vi "PH_Beamline.panel.vi"(0 "object ref":refnum<vi>, 5 "error in (no error)":errorcluster) -> (19 "error out":errorcluster)   [LabVIEW 2014, in "PH_Beamline.lvlib"]
doc: "By this VI a hardware switch can be monitored and switched. \n\nThe indicators \"FALSE\", \"TRUE\" and \"SWITCH STATE\" show the value of the Beckhoff-Tag: blue indicates bad tag status reference problems, darkgreen false and lightgreen true. If everything is working fine, \"FALSE\" and \"SWITCH STATE\" should show the same value, while \"TRUE\" has the opposite value. The caption of the sensors for \"FALSE\" and \"TRUE\" are taken out of the database. In case of only one or no sensor these GUI elements are not shown at all.\n\nThe oval button switches. It should be in the same state as the \"SWITCH STATE\" indicator. \n\n\"Delete Instance\" disconnects and removes the instance from the PCS.\n\n\nLicense Agreement for this software:\n\nCopyright (C)\nGesellschaft für Schwerionenforschung, GSI\nPlanckstr. 1\n64291 Darmstadt\nGermany\n\nContact: D.Beck@gsi.de \n\nThis program is free software; you can redistribute it and/or modify it under the terms of the GNU General Public License as published by the Free Software Foundation; either version 2 of the license, or (at your option) any later version.\n\nThis program is distributed in the hope that it will be useful, but WITHOUT ANYW ARRANTY; without even the implied warranty of MERCHANTABILITY or FITNESS FOR A PARTICULAR PURPOSE. See the GNU General License for more details (http://www.gnu.org).\n\nGesellschaft für Schwerionenforschung, GSI\nPlanckstr. 1, 64291 Darmstadt, Germany\nFor all questions and ideas contact: M.Richter@gsi.de, H.Brand@gsi.de or D.Beck@gsi.de.\nLast update: 18-DEC-2002"
uses:
  PH_Beamline.lvlib
  PH_Basics/PH_Common/Picture/PH_Picture.GUI Element 48x48.ctl
  PH_Basics/PH_Common/Picture/PH_Picture.GUI Element 36x36.ctl
  PH_Basics/PH_Common/Picture/PH_Picture.GUI Element 24x36.ctl
  PH_Basics/PH_Common/Picture/PH_Picture.GUI Element.ctl
  PH_Basics/PH_Common/Picture/PH_Picture.GUI Element 36x24.ctl
  PH_Basics/PH_Common/Picture/PH_Picture.GUI Element 60x12.ctl
  PH_Basics/PH_Common/Picture/PH_Picture.GUI Element 12x60.ctl
  PH_Beamline.Operation Mode.ctl
  PH_Beamline.Switch Instances.ctl
  PH_Beamline.6P Switch Instances.ctl
  PH_Beamline.Black Box Instances.ctl
  PH_Beamline.Switch GUI Instances.ctl
  PH_Beamline.Switch+6P Instances.ctl
  PH_Beamline.Force Sensor Instances.ctl
  PH_Basics/PH_SystemInformation/PH_SystemInformation.GUI Refs.ctl
  PH_BL-Master/PH_BL-Master.GUI Refs.ctl
  PH_Beamline.GUI Refs.ctl
  PH_Beamline.Motion GUI Instances.ctl
  PH_Basics/PH_StatusHandler/PH_StatusHandler.Status.ctl
  CS_Core/CSObj/CSObj.lvlib
  PH_Basics/PH_StatusHandler/PH_StatusHandler.lvlib
  PH_Basics/PH_Common/PH_Common.lvlib
  PH_Classes/PH_Switch/PH_Switch.lvlib
  PH_Motion/PH_Sixpack_Switch/PH_Sixpack_Switch.lvlib
  PH_Classes/PH_BlackBox/PH_BlackBox.lvlib
  PH_BL-Master/PH_BL-Master.lvlib
  PH_Basics/PH_SystemInformation/PH_SystemInformation.lvlib
  PH_Basics/PH_Class/PH_Class.lvlib
panel:
  in  "Force Sensor Instances":T1="MM1_ForceSensor"
  in  "Compressor_Turnbox_1_Trans_6PGUI":T2
  in  "Compressor_Turnbox_1_6PGUI":T3
  in  "Compressor_Turnbox_2_Trans_6PGUI":T2
  in  "Compressor_Turnbox_2_6PGUI":T3
  in  "Experiment_Targetmanipulator_6PGUI":T3
  in  "Experiment_Targetmanipulator_TRANS_6PGUI":T4
  in  "Experiment_Targetmanipulator_TURN_6PGUI":T3
  in  "Switch and 6P Instances":T5="BL_Position_MM5::MA_MM5_6PGUI"
  in  "Switch GUI Instances":T6="Shutter_Exp_Laserbay_Interlock"
  in  "Black Box Instances":T7="PA_CH1_BB"
  in  "6P Switch Instances":T8="COS_Sensitivity_Switch"
  in  "Switch Instances":T9="MA01_CH1"
  out "Exp.-Shutters closed":bool
  in  "Remote Desktop Connection":bool
  out "PHELIX_Beckhoff_Watchdog":bool caption="Failure Beckhoff"
  out "PHELIX_Timing_Mode":enum32{"10 Hz", "0.5 Hz", "Shot"}(radio) caption="Modeselector"
  out "Emergency Off":u32(colorbox)
  out "Igni FR: Heating off":bool
  out "Igni MA 5: Heating off":bool
  out "Igni MA 4: Heating off":bool
  out "Igni MA 3: Heating off":bool
  out "Igni MA 2: Heating off":bool
  out "Igni MA 1: Heating off":bool
  in  "Z6 Main":bool
  in  "PCS Main":bool
  in  "PCS System Indicator":bool
  in  "CoG":bool
  in  "Calibrator":bool
  in  "Image Statistician":bool
  out "Shutter_Exp3":bool=TRUE
  out "Shutter_Exp2":bool=TRUE
  out "Shutter_Exp1":bool=TRUE
  out "Shutter Exp 4 (Z6)":u32(colorbox)
  out "Shutter Exp 3":u32(colorbox)
  out "Shutter Exp 2":u32(colorbox)
  out "Shutter Exp 1":u32(colorbox)
  in  "Tab Control":T10(tab)=enum."In.-Box"
  in  "\"D:\\PCS\\Remote Access\\ns.rdp\"":bool caption="OK Button"
  out "ns Frontend ok":bool caption="ok"
  in  "ns_WP_RR_6PWpGUI":T11
  in  "Hop 15":bool
  out "BL ns 8":u32(colorbox)
  in  "NS_Shut_PA_BB":bool=TRUE
  out "BL ns 7":u32(colorbox)
  out "BL ns 6":u32(colorbox)
  out "BL ns 5":u32(colorbox)
  out "BL ns 4":u32(colorbox)
  out "BL ns 3":u32(colorbox)
  out "BL ns 2":u32(colorbox)
  out "BL ns 1":u32(colorbox)
  in  "ns_Nearfield_Ring_Exit_ImageOperator":bool=TRUE
  in  "ns_Nearfield_Ring_Exit_Cam":bool=TRUE
  in  "ns_Farfield_Ring_Exit_ImageOperator":bool=TRUE
  in  "ns_Farfield_Ring_Exit_Cam":bool=TRUE
  in  "ns_Exit_Powermeter":bool=TRUE
  in  "Hop 23":bool
  in  "\"D:\\PCS\\Remote Access\\fs.rdp\"":bool caption="OK Button"
  out "fs Frontend ok":bool caption="ok"
  out "BL fs 17":u32(colorbox)
  out "BL fs 16":u32(colorbox)
  in  "YLF_WP_6PWpGUI":T12
  in  "fs_WP_Exit_6PWpGUI":T11
  in  "fs_OO_Spectrometer":bool=TRUE
  out "BL fs 8":u32(colorbox)
  out "BL fs 10":u32(colorbox)
  in  "fs_RR_Cavity_NF2GUI":T3
  in  "fs_Stretcher_6PGUI":T3
  out "BL fs 15":u32(colorbox)
  in  "FS_Shut_PA_BB":bool=TRUE
  out "BL fs 14":u32(colorbox)
  in  "Hop 3":bool
  out "BL fs 13":u32(colorbox)
  in  "FS_Switch_YLF_BB":T3
  out "BL fs 12":u32(colorbox)
  out "BL fs 11":u32(colorbox)
  out "BL fs 7":u32(colorbox)
  out "BL fs 5":u32(colorbox)
  out "BL fs 9":u32(colorbox)
  out "BL fs 6":u32(colorbox)
  out "BL fs 4":u32(colorbox)
  out "BL fs 3":u32(colorbox)
  out "BL fs 2":u32(colorbox)
  out "BL fs 1":u32(colorbox)
  in  "fs_Nearfield_Frontend_ImageOperator":bool=TRUE
  in  "fs_Nearfield_Frontend_Cam":bool=TRUE caption="fs NF Exit Cam"
  in  "fs_Synchrolock_Watch":bool=TRUE
  out "uOPA ok":bool caption="ok"
  in  "\"D:\\PCS\\Remote Access\\uOPA.rdp\"":bool caption="OK Button"
  out "BL uOPA 9":u32(colorbox)
  in  "uOPA_Pump_OO_Spectrometer":bool=TRUE
  in  "uOPA_Pump_WP_6PWpGUI":T11
  out "BL uOPA 8":u32(colorbox)=6618880
  out "BL uOPA 7":u32(colorbox)
  out "BL uOPA 6":u32(colorbox)
  out "BL uOPA 5":u32(colorbox)
  out "BL uOPA 4":u32(colorbox)
  out "BL uOPA 3":u32(colorbox)
  out "BL uOPA 2":u32(colorbox)
  out "BL uOPA 1":u32(colorbox)
  out "BL uOPA 0":u32(colorbox)
  in  "Hop 24":bool
  in  "uOPA_Regen_Cam":bool=TRUE
  in  "uOPA_Pump_Powermeter":bool=TRUE
  in  "PA_SHS_Input_Cam":bool=TRUE
  in  "PA_CH1_BB":T13 caption="CH"
  out "BL PA 21":u32(colorbox)
  out "PA_Bypass_In":T3
  out "BL PA 24":u32(colorbox)
  out "BL PA 23":u32(colorbox)
  in  "PA_delayed_BB":bool=TRUE
  in  "PA_Input_2_Beam_6PWpGUI":T11
  out "BL PA 11":u32(colorbox)
  in  "PA_ML_T3_Exit_6P4QGUI":T11 caption="PA Lens"
  in  "PA_SA_6P4QGUI":T3
  out "BL PA 4":u32(colorbox)
  in  "PA_Input_Delay_6PGUI":T3
  out "BL PA 8":u32(colorbox)
  out "BL PA 7":u32(colorbox)
  out "BL PA 6":u32(colorbox)
  out "BL PA 5":u32(colorbox)
  out "BL PA 3":u32(colorbox)
  in  "PA_non_delayed_BB":bool=TRUE
  in  "PA-Backreflection-Meas":bool=TRUE
  in  "PA_PC_WP_2_BB":bool=TRUE
  in  "Hop 22":bool
  in  "Hop 16":bool
  out "BL PA 20":u32(colorbox)
  in  "PA_PC_WP_BB":bool=TRUE
  in  "PA_PiH_VSF2_6PGUI":T11
  out "BL PA 10":u32(colorbox)
  in  "PA_Shut_Input_BB":bool=TRUE
  in  "PA_PiH_VSF4_6PGUI":T11
  in  "Hop 6":bool
  in  "Hop 5":bool
  in  "Hop 4":bool
  in  "PA_MM_P_Input_NF2GUI":T3
  in  "PA_MM_C_Input_NF2GUI":T3
  out "BL PA 0":u32(colorbox)
  out "BL PA 16":u32(colorbox)
  out "BL PA 12":u32(colorbox)
  out "BL PA 14":u32(colorbox)
  out "PA_VacuumControl::PA_VacuumControl_Telescope 2":dbl=2000.0 caption="mbar" format="%#_2e"
  out "PA_VacuumControl::PA_VacuumControl_Telescope 3":dbl=2000.0 caption="mbar" format="%#_2e"
  out "PA_VacuumControl::PA_VacuumControl_Telescope 4":dbl=2000.0 caption="mbar" format="%#_2e"
  out "PA_VacuumControl::PA_VacuumControl_Bridge":dbl=2000.0 caption="mbar" format="%#_2e"
  out "BL PA 18":u32(colorbox)
  out "PA_Bypass_Out":T3
  out "BL PA 22":u32(colorbox)
  in  "PA_Switch_Lab_BB":T3
  in  "PA_Exit_Shut_BB":bool=TRUE
  out "BL PA 19":u32(colorbox)
  out "BL PA 15":u32(colorbox)
  out "BL PA 13":u32(colorbox)
  in  "PA_Nearfield_Input_ImageOperator":bool=TRUE
  in  "PA_Nearfield_Input_Cam":bool=TRUE
  in  "PA_Farfield_Input_ImageOperator":bool=TRUE
  in  "PA_Farfield_Input_Cam":bool=TRUE
  out "BL PA 9":u32(colorbox)
  out "BL PA 1":u32(colorbox)
  out "PA_VacuumControl::PA_VacuumControl_Telescope 1":dbl=2000.0 caption="mbar" format="%#_2e"
  out "PA_VacuumControl::PA_VacuumControl_PA global":dbl=2000.0 caption="mbar" format="%#_2e"
  out "BL PA 2":u32(colorbox)
  out "BL PA 17":u32(colorbox)
  out "PreAmp ok":bool caption="ok"
  in  "\"D:\\PCS\\Remote Access\\PA-Input.rdp\"":bool caption="OK Button"
  out "PA ED ok":bool caption="ok"
  in  "\"D:\\PCS\\Remote Access\\PA-Exit.rdp\"":bool caption="OK Button"
  in  "PA_SHS_Exit_Cam":bool=TRUE
  in  "PA_ED_FILT1_BB":bool=TRUE
  in  "Hop 7":bool
  in  "PA_Exit_Powermeter":bool=TRUE
  out "BL PA ED 2":u32(colorbox)
  in  "PA_WP_Exit_6PWpGUI":T12
  in  "PA_Farfield_Exit_ImageOperator":bool=TRUE
  in  "PA_Farfield_Exit_Cam":bool=TRUE caption="PA FF Exit Cam"
  in  "PA_Nearfield_Exit_ImageOperator":bool=TRUE
  in  "PA_Nearfield_Exit_Cam":bool=TRUE caption="PA NF Exit Cam"
  in  "PA_ED_FILT2_BB":T12 caption="Filt 2"
  out "BL PA ED 1":u32(colorbox)
  in  "MA_ML_In_6P4QGUI":T11 caption="PA Lens"
  in  "PA_Bridge_CH_Input_MA_BB":T13 caption="CH"
  out "BL MA-IB 9":u32(colorbox)
  out "BL MA-IB 8":u32(colorbox)
  out "BL MA-IB 14":u32(colorbox)
  out "BL MA-IB 12":u32(colorbox)
  out "BL MA-IB 13":u32(colorbox)
  in  "MA_Nearfield_PiH_out_ImageOperator":bool=TRUE
  in  "MA_Nearfield_PiH_out_Cam":bool=TRUE
  in  "MA_InB_IM_Out_Switch":T3
  in  "MA_InB_DP_Out_Switch":bool=TRUE
  in  "MA_InB_DP_In_Switch":bool=TRUE
  out "BL MA-IB 11":u32(colorbox)
  out "BL MA-IB 10":u32(colorbox)
  in  "MA_InB_IM_In_Switch":T3
  out "BL MA-IB 7":u32(colorbox)
  out "BL MA-IB 6":u32(colorbox)
  out "BL MA-IB 5":u32(colorbox)
  in  "MA_Diffusor_Inject_In_BB":bool=TRUE
  out "BL MA-IB 4":u32(colorbox)
  out "BL MA-IB 3":u32(colorbox)
  out "BL MA-IB 2":u32(colorbox)
  out "BL MA-IB 1":u32(colorbox)
  in  "PA_C_MA_6PGUI":T3
  in  "MA_Inject_In_ImageOperator":bool=TRUE
  in  "MA_Inject_In_Cam":bool=TRUE
  in  "MA_Inject_P_6PGUI":T3
  in  "Hop 2":bool
  in  "Hop 1":bool
  in  "MA_Nearfield_PiH_in_ImageOperator":bool=TRUE
  in  "MA_Nearfield_PiH_in_Cam":bool=TRUE
  in  "MA_Inject_C_NF2GUI":T3
  out "MA_IB_Ready":bool
  in  "PA_MA_Bridge_Input_Cam":bool=TRUE
  in  "\"D:\\PCS\\Remote Access\\MA.rdp\"":bool caption="OK Button"
  out "In.-Box ok":bool caption="ok"
  in  "\"D:\\PCS\\Remote Access\\MA.rdp\" 2":bool caption="OK Button"
  in  "FR+MT_Flowbox_off":bool caption="Flowboxes FR + MT off"
  in  "MainAmp_Flowbox_off":bool caption="Flowboxes MA off"
  out "MainAmp ok":bool caption="ok"
  in  "MM1_ForceSensor":bool
  in  "MA01_CH1":T13 caption="CH"
  in  "MA01_CH2":T13 caption="CH"
  in  "MA01_CH4":T13 caption="CH"
  in  "MA01_CH3":T13 caption="CH"
  out "BL MA 3":u32(colorbox)
  out "BL MA 9":u32(colorbox)
  in  "Hop 11":bool
  out "BL MA 8":u32(colorbox)
  in  "MA_Shut_AlignCam_BB":bool=TRUE
  out "MA01_O2_Beamline_MM3":dbl=99.0 caption="%O2" format="%#_2f"
  out "MA01_O2_Beamline_MM1":dbl=99.0 caption="%O2" format="%#_2f"
  in  "Hop 9":bool
  in  "Hop 8":bool
  in  "MA_Alignment_ImageOperator":bool=TRUE
  in  "MA_Alignment_Cam":bool=TRUE
  out "BL MA 7":u32(colorbox)
  out "BL MA 2":u32(colorbox)
  out "MA_VacuumControl::MA_VacuumControl_MA Telescope Prepressure":dbl=2000.0 caption="mbar" format="%#_6e"
  out "BL MA 6":u32(colorbox)
  out "BL MA 5":u32(colorbox)
  out "BL MA 4":u32(colorbox)
  out "BL MA 1":u32(colorbox)
  out "MA_VacuumControl::MA_VacuumControl_MA Telescope":dbl=2000.0 caption="mbar" format="%#_6e"
  in  "MA_MM3_6PGUI":T14
  in  "MA_MM4_6PGUI":T14
  in  "MA_MM2_6PGUI":T14
  in  "MA_MM1_6P4QGUI":T14
  in  "MA_MM1_Bend_6P4QGUI":T14
  in  "\"D:\\PCS\\Remote Access\\MAS.rdp\"":bool caption="OK Button"
  out "MAS ok":bool caption="ok"
  in  "MAS_SHS_Cam":bool=TRUE
  in  "MAS_FF_HamamatsuCam":bool=TRUE
  in  "MAS_Attenuator_3_BB":T12
  in  "MAS_Attenuator_2_BB":T12
  in  "MAS_OO_Spectrometer":bool=TRUE
  in  "MAS_Discrete_Spectro_Rev6PGUI":T11
  out "BL MAS 3":u32(colorbox)
  in  "Hop 10":bool
  in  "MAS_Beam_Fine_Attenuator_6PWpGUI":T11
  in  "MAS_Farfield_High_Res_ImageOperator":bool=TRUE
  in  "MAS_Farfield_High_Res_Cam":bool=TRUE
  out "BL MAS 5":u32(colorbox)
  in  "MAS_Nearfield_ImageOperator":bool=TRUE
  in  "MAS_Nearfield_Cam":bool=TRUE
  out "BL MAS 4":u32(colorbox)
  in  "MAS_Attenuator_1_BB":bool=TRUE
  out "BL MAS 2":u32(colorbox)
  in  "MAS_Powermeter":bool=TRUE
  out "BL MAS 1":u32(colorbox)
  out "Booster ok":bool caption="ok"
  out "BL Boo 5":u32(colorbox)
  in  "Hop 17":bool
  in  "MA_MM8_6PGUI":T3
  in  "Hop 13":bool
  out "BL Boo 4":u32(colorbox)
  in  "Hop 12":bool
  out "BL Boo 3":u32(colorbox)
  out "BL Boo 2":u32(colorbox)
  out "BL Boo 1":u32(colorbox)
  in  "BL_Position_MM5::MA_MM5_6PGUI":T3
  in  "Calorimeter_Switch":bool=TRUE
  in  "\"D:\\PCS\\Remote Access\\COS.rdp\"":bool caption="OK Button"
  out "Compressor ok":bool caption="ok"
  in  "Compressor_Grating_1_6PGUI":T2
  in  "Compressor_Grating_2_6PGUI":T2
  in  "COS_Filt1_BB":bool=TRUE
  in  "COS-SSAC":bool=TRUE
  in  "COS_SSAC_Cam":bool=TRUE
  in  "COS_WP_6PWpGUI":T11
  in  "COS_Filt2_BB":T11 caption="Filt 2"
  out "BL Compressor 8":u32(colorbox)
  in  "COS_Sensitivity_Switch":bool=TRUE
  in  "COS_NF_Cam":bool=TRUE
  in  "COS_FF_Cam":bool=TRUE
  out "Compressor_VacuumControl::Compressor_VacuumControl_Compressor Pre":dbl=2000.0 caption="mbar" format="%#_6e"
  out "Compressor_VacuumControl::Compressor_VacuumControl_Compressor":dbl=2000.0 caption="mbar" format="%#_6e"
  out "BL Compressor 5":u32(colorbox)
  out "BL Compressor 6":u32(colorbox)
  out "BL Compressor 7":u32(colorbox)
  in  "Compressor_LM_6PGUI":T3
  out "BL Compressor 4":u32(colorbox)
  out "BL Compressor 2":u32(colorbox)
  out "BL Compressor":u32(colorbox)
  in  "Compressor_Grating_1_Tip+Tilt_6PGUI":T3
  in  "Compressor_Grating_2_Tip+Tilt_6PGUI":T3
  in  "Hop 19":bool
  in  "Hop 20":bool
  out "BL Compressor 3":u32(colorbox)
  out "Vacuum no shotcond Comp LB":bool caption="Vacuum is no shot condition!"
  in  "\"D:\\PCS\\Remote Access\\Experiment.rdp\"":bool caption="OK Button"
  out "Intensity LB below Limit":bool caption="I < 1E18W/cm²"
  out "HV room locked?":i32(ring) caption="Enabling State" items=["no info", "HV room open", "HV room locked"]
  in  "Shutter_Exp_Laserbay_Interlock":bool caption="request Light"
  out "Laserbay evacuated?":i32(ring) caption="Enabling State" items=["no info", "LB not evacuated", "LB evacuated"]
  out "Exp: Shotmode":T15 caption="Enabling State" items=["no info", "no Shotmode", "Shotmode"]
  out "Experiment LB ok":bool caption="ok"
  out "BL Exp LB 8":u32(colorbox)
  out "BL Exp LB 7":u32(colorbox)
  out "BL Exp LB 6":u32(colorbox)
  out "Windowshutter_TB3_Watch":bool=TRUE
  out "Experiment_VacuumControl::Experiment_VacuumControl_Experiment Pirani":dbl=2000.0 caption="mbar" format="%#_6e"
  out "Experiment_VacuumControl::Experiment_VacuumControl_Experiment":dbl=2000.0 caption="mbar" format="%#_6e"
  out "Windowshutter_TB2_Watch":bool=TRUE
  out "BL Exp LB 5":u32(colorbox)
  out "BL Exp LB 4":u32(colorbox)
  in  "Shutter_Exp_Laserbay":bool=TRUE
  in  "Hop 18":bool
  out "BL Exp LB 3":u32(colorbox)
  out "BL Exp LB":u32(colorbox)
  out "BL Exp LB 2":u32(colorbox)
  out "MA_VacuumControl::MA_VacuumControl_Z6 Telescope BL Prepressure":dbl=2000.0 caption="mbar" format="%#_2e"
  out "Shutter_Exp4":bool=TRUE
  in  "BL-Z6-CH9":T13 caption="CH"
  in  "Z6 Beamline":bool
  out "BL MT 4":u32(colorbox)
  out "MA_VacuumControl::MA_VacuumControl_Z6 Telescope BL":dbl=2000.0 caption="mbar" format="%#_2e"
  in  "Hop 14":bool
  out "BL MT 3":u32(colorbox)
  out "BL MT 2":u32(colorbox)
  out "BL MT 1":u32(colorbox)
  in  "MA_MM9_6PGUI":T3
  in  "BL-Z6-Beamdump":bool=TRUE
  out "Mirrortower ok":bool caption="ok"
  out "Laserlab ok":bool caption="ok"
  in  "\"D:\\PCS\\Remote Access\\Laserlabor.rdp\"":bool caption="OK Button"
  in  "LL_Comp_FF_Cam":bool=TRUE
  in  "LL-SSAC":bool=TRUE
  in  "LL_SSAC_Cam":bool=TRUE
  out "BL LL 14":u32(colorbox)
  in  "LL_Shut_Comp_Output_BB":bool=TRUE
  in  "LL_Comp_Input_Cam":bool=TRUE caption="fs NF Exit Cam"
  out "BL LL 13":u32(colorbox)
  out "BL LL 12":u32(colorbox)
  in  "LL_Comp_Length_6PGUI":T4
  in  "LL_Comp_Grating_Rot_6PGUI":T3
  in  "LL_Shut_Comp_FF_BB":bool=TRUE
  out "BL LL 11":u32(colorbox)
  in  "LL_Shut_Comp_Input_BB":bool=TRUE
  out "BL LL 10":u32(colorbox)
  out "BL LL 9":u32(colorbox)
  in  "LL_Comp_P_6PGUI":T3
  out "BL LL 8":u32(colorbox)
  in  "LL_Comp_C_6PGUI":T3
  out "BL LL 7":u32(colorbox)
  out "BL LL 6":u32(colorbox)
  in  "PA_LL_CH_Output_BB":bool=TRUE
  in  "PA_LL_Output_Cam":bool=TRUE caption="PA NF Exit Cam"
  out "Intensity LL below Limit":bool caption="I < 1E18W/cm²"
  out "BL LL 5":u32(colorbox)
  in  "PA_LL_CH_Input_BB":bool=TRUE
  out "BL LL 4":u32(colorbox)
  out "BL LL 3":u32(colorbox)
  out "BL LL 2":u32(colorbox)
  in  "PA_LL_P_6PGUI":T3
  in  "PA_LL_C_6PGUI":T3
  in  "Shutter_Laserlab_Interlock":bool caption="request Light"
  out "BL LL 1":u32(colorbox)
  out "BL LL 0":u32(colorbox)
  in  "Hop 21":bool
  in  "Shutter_Laserlab":bool=TRUE
  out "Laserlab evacuated?":i32(ring) caption="Enabling State" items=["no info", "LL not evacuated", "LL evacuated"]
  out "LL: Shotmode":T15 caption="Enabling State" items=["no info", "no Shotmode", "Shotmode"]
  in  "PA_LL_Input_Cam":bool=TRUE caption="PA FF Exit Cam"
  out "Ready for Shot":bool
  out "MainAmp enabled":u32(colorbox)
  out "Laser enabled":u32(colorbox)
  out "PreAmp enabled":u32(colorbox)
  in  "Minimize":bool
  in  "Delete":bool
  # "PCS"
  # "3.40"
  # "Stretcher"
  # "PL8000"
  # "PL9000"
  # "YLF"
  # "MIRA"
  # "Lin Regen"
  # "Ring  Regen"
  # "Verdi"
  # "Fiber Amplifier"
  # "Regen"
  # "SHS"
  # "19 DP"
  # "45 DP"
  # "2"
  # "1"
  # "SHS"
  # "MM3"
  # "1"
  # "2"
  # "3"
  # "SHS"
  # "H"
  # "2"
  # "1"
  # "Laserbay          Laserlab"
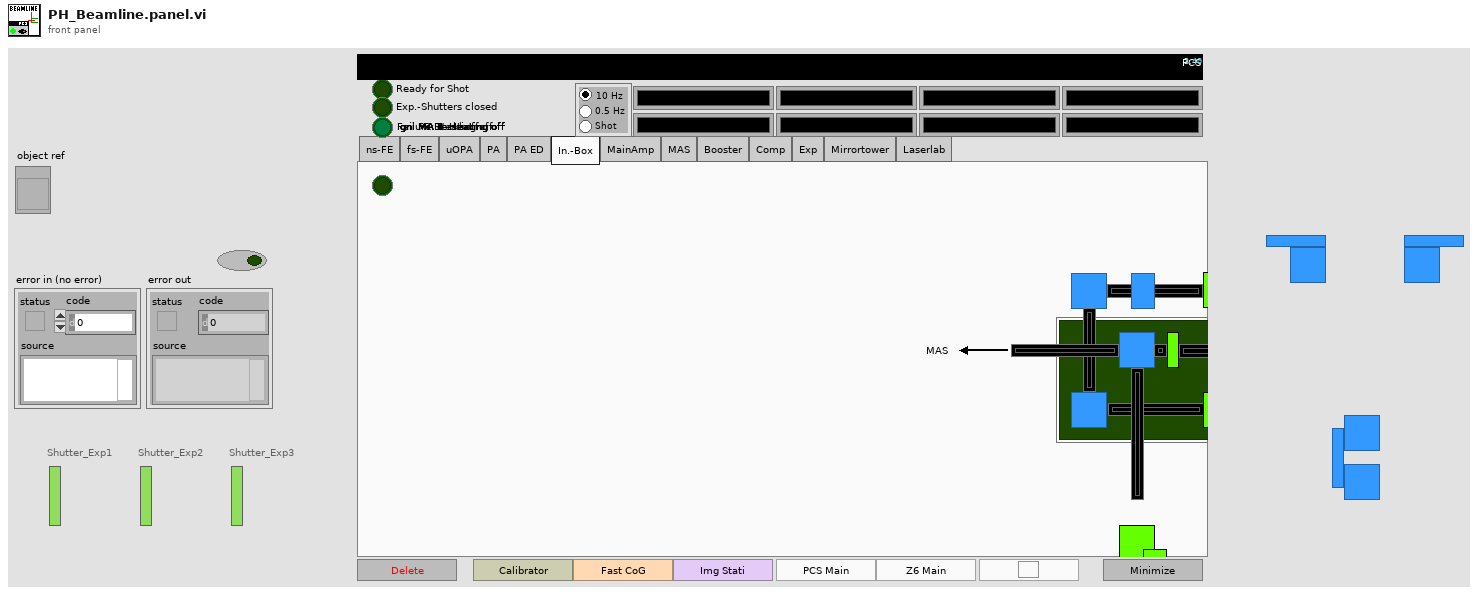
[diagram p1: front panel]
types:
  T1 = typedef "PH_Beamline.lvlib/PH_Beamline.Force Sensor Instances.ctl" = string
  T2 = typedef "PH_Common.lvlib/PH_Picture.GUI Element 60x12.ctl" = picture
  T3 = typedef "PH_Common.lvlib/PH_Picture.GUI Element 36x36.ctl" = picture
  T4 = typedef "PH_Common.lvlib/PH_Picture.GUI Element 12x60.ctl" = picture
  T5 = typedef "PH_Beamline.lvlib/PH_Beamline.Switch+6P Instances.ctl" = string
  T6 = typedef "PH_Beamline.lvlib/PH_Beamline.Switch GUI Instances.ctl" = string
  T7 = typedef "PH_Beamline.lvlib/PH_Beamline.Black Box Instances.ctl" = string
  T8 = typedef "PH_Beamline.lvlib/PH_Beamline.6P Switch Instances.ctl" = string
  T9 = typedef "PH_Beamline.lvlib/PH_Beamline.Switch Instances.ctl" = string
  T10 = enum32{"ns-FE", "fs-FE", "uOPA", "PA", "PA ED", "In.-Box", "MainAmp", "MAS", "Booster", "Comp", "Exp", "Mirrortower", "Laserlab"}
  T11 = typedef "PH_Common.lvlib/PH_Picture.GUI Element 24x36.ctl" = picture
  T12 = typedef "PH_Common.lvlib/PH_Picture.GUI Element 36x24.ctl" = picture
  T13 = typedef "PH_Common.lvlib/PH_Picture.GUI Element.ctl" = picture
  T14 = typedef "PH_Common.lvlib/PH_Picture.GUI Element 48x48.ctl" = picture
  T15 = typedef "PH_Beamline.lvlib/PH_Beamline.Operation Mode.ctl" = i32
  T16 = typedef "PH_Beamline.lvlib/PH_Beamline.GUI Refs.ctl" = cluster{"Vision on this Node?":bool, "Vision Knobs":refnum<vi>[], "GUI Refs":cluster{"PA ok":refnum<vi>, "MA ok":refnum<vi>, "fs FE ok":refnum<vi>, "ns FE ok":refnum<vi>, "PA ED ok":refnum<vi>, "MAS ok":refnum<vi>, "Booster ok":refnum<vi>, "Mirrortower ok":refnum<vi>, "In.-Box ok":refnum<vi>, "Compressor ok":refnum<vi>, "Experiment LB ok":refnum<vi>, "Experiment LL ok":refnum<vi>, "PHELIX_Beckhoff_Watchdog":refnum<vi>, "Shutters closed":refnum<vi>, "uOPA ok":refnum<vi>, "Vacuum no shotcond Comp LB":refnum<vi>}, "PP Igni Heating GUI Refs":refnum<vi>[], "Refs BL PA":cluster{"undelayed Line before Shutter":refnum<vi>[], "undelayed Line after Shutter":refnum<vi>[], "before Bypass":refnum<vi>[], "delayed Line before Shutter":refnum<vi>[], "delayed Line after Shutter":refnum<vi>[], "before Shutter Input":refnum<vi>[], "after Shutter Input":refnum<vi>[], "Bypass":refnum<vi>[], "before Shutter Exit":refnum<vi>[], "after Shutter Exit":refnum<vi>[], "to MA":refnum<vi>[], "to Lab":refnum<vi>[]}, "Refs BL MA":refnum<vi>[], "Refs BL MA-IB":refnum<vi>[], "Refs BL fs":refnum<vi>[], "Refs BL PA ED":refnum<vi>[], "Refs BL MAS":refnum<vi>[], "Refs BL Boo":refnum<vi>[], "Refs BL ns":refnum<vi>[], "Refs BL Mirrortower":refnum<vi>[], "Refs BL Compressor":refnum<vi>[], "Refs BL Exp LB":refnum<vi>[], "Refs BL LL":refnum<vi>[], "Refs BL uOPA":refnum<vi>[], "Ref Op Mode Exp LB":refnum<vi>, "Ref Laserbay evacuated":refnum<vi>, "Ref Op Mode Exp LL":refnum<vi>, "Ref Laserlab evacuated":refnum<vi>, "Ref HV room locked":refnum<vi>, "Ref Bridge LB":refnum<vi>, "Ref Bridge LL":refnum<vi>}
  T17 = typedef "PH_BL-Master.lvlib/PH_BL-Master.GUI Refs.ctl" = cluster{"Vac GUI Refs":refnum<vi>[], "O2 GUI Refs":refnum<vi>[], "Ready for Shot":refnum<vi>, "Boolean Condition Service Subscriber GUI Refs":refnum<vi>[], "Vision ID on same Node":string, "Picture Condition Service Subscriber GUI Refs":refnum<vi>[], "6P 4Q GUI Refs":refnum<vi>[], "Ref Switch GUI Instances":refnum<vi>, "Ref 6P Switch Instances":refnum<vi>, "Ref BB Instances":refnum<vi>, "Ref Switch Instances":refnum<vi>, "Ref Switch and 6P State Instances":refnum<vi>, "Boolean Status Service Subscriber GUI Refs":refnum<vi>[], "Picture Status Service Subscriber GUI Refs":refnum<vi>[], "Force Sensor Instances":refnum<vi>, "GUI Ref Delete":refnum<vi>}
  T18 = typedef "PH_SystemInformation.lvlib/PH_SystemInformation.GUI Refs.ctl" = cluster{"Laser":refnum<vi>, "PreAmp":refnum<vi>, "MainAmp":refnum<vi>, "Emergency Off":refnum<vi>, "Exp 1":refnum<vi>, "Exp 2":refnum<vi>, "Exp 3":refnum<vi>, "Exp 4":refnum<vi>, "Timing Mode GUI Ref":refnum<vi>}
  T19 = cluster{"undelayed Line before Shutter":refnum<vi>[], "undelayed Line after Shutter":refnum<vi>[], "before Bypass":refnum<vi>[], "delayed Line before Shutter":refnum<vi>[], "delayed Line after Shutter":refnum<vi>[], "before Shutter Input":refnum<vi>[], "after Shutter Input":refnum<vi>[], "Bypass":refnum<vi>[], "before Shutter Exit":refnum<vi>[], "after Shutter Exit":refnum<vi>[], "to MA":refnum<vi>[], "to Lab":refnum<vi>[]}
  T20 = typedef "PH_Beamline.lvlib/PH_Beamline.Motion GUI Instances.ctl" = string
  T21 = enum16{"None", "PCS Main", "Z6 Main", "PCS Beamline", "Z6 Beamline", "Image Statistician", "Powermeter Statistician", "SHS Anal Statistician", "Image Center of Gravity", "Image Calibrator", "SHS Analysis Calibrator", "Cam List", "Powermeterlist", "6P List", "BB List", "Switch List", "Sequence Watch"}
  T22 = typedef "PH_Beamline.lvlib/PH_Beamline.i attribute.ctl" = cluster{"GUI Refs":cluster{"PA ok":refnum<vi>, "MA ok":refnum<vi>, "fs FE ok":refnum<vi>, "ns FE ok":refnum<vi>, "PA ED ok":refnum<vi>, "MAS ok":refnum<vi>, "Booster ok":refnum<vi>, "Mirrortower ok":refnum<vi>, "In.-Box ok":refnum<vi>, "Compressor ok":refnum<vi>, "Experiment LB ok":refnum<vi>, "Experiment LL ok":refnum<vi>, "PHELIX_Beckhoff_Watchdog":refnum<vi>, "Shutters closed":refnum<vi>, "uOPA ok":refnum<vi>, "Vacuum no shotcond Comp LB":refnum<vi>}, "Refs BL MA":refnum<vi>[], "Refs BL MA-IB":refnum<vi>[], "Refs BL fs":refnum<vi>[], "Refs BL PA ED":refnum<vi>[], "Refs BL MAS":refnum<vi>[], "Refs BL Boo":refnum<vi>[], "Refs BL ns":refnum<vi>[], "Refs BL Mirrortower":refnum<vi>[], "Refs BL Compressor":refnum<vi>[], "Refs BL Exp LB":refnum<vi>[], "Radiation Safety":cluster{"Exp Laserbay":cluster{"Ref Op Mode":refnum<vi>, "Ref Laserbay evacuated":refnum<vi>, "Tagname LB evacuated":string, "Shot Mode":T15, "Laserbay evacuated?":i32, "Tagname HV room locked":string, "HV room locked?":i32, "Ref HV room locked":refnum<vi>, "Tagname bridged?":string, "Ref Bridge":refnum<vi>, "I<1E18W/cm²":bool}, "Exp Laserlab":cluster{"Ref Op Mode":refnum<vi>, "Ref Laserlab evacuated":refnum<vi>, "Tagname LL evacuated":string, "Shot Mode":T15, "Laserlab evacuated?":i32, "Tagname bridged?":string, "Ref Bridge":refnum<vi>, "I<1E18W/cm²":bool}}, "Refs BL LL":refnum<vi>[], "PP Igni Heating GUI Refs":refnum<vi>[], "PP Igni Heating Tagnames ":string[], "Refs BL PA":cluster{"undelayed Line before Shutter":refnum<vi>[], "undelayed Line after Shutter":refnum<vi>[], "before Bypass":refnum<vi>[], "delayed Line before Shutter":refnum<vi>[], "delayed Line after Shutter":refnum<vi>[], "before Shutter Input":refnum<vi>[], "after Shutter Input":refnum<vi>[], "Bypass":refnum<vi>[], "before Shutter Exit":refnum<vi>[], "after Shutter Exit":refnum<vi>[], "to MA":refnum<vi>[], "to Lab":refnum<vi>[]}, "BL":cluster{"YLF_BL_Status":i32, "fs_BL_Status":i32, "fs_YLF_BL_Status":i32, "ns_BL_Status":i32, "PA_Input_BL_Status":i32, "PA_UnDelay_BL_Status":i32, "PA_Delay_BL_Status":i32, "PA_BL_Status":i32, "PA_Bypass_BL_Status":i32, "PA_Exit_BL_Status":i32, "PA_LL_BL_Status":i32, "LL_BL_Status":i32, "PA_MA_BL_Status":i32, "MA_Exit_BL_Status":i32, "MA_Z6_BL_Status":i32, "Z6_BL_Status":i32, "MA_LB_BL_Status":i32, "LB_TB2_BL_Status":i32, "PA_before_Bypass_BL_Status":i32, "LB_TB3_BL_Status":i32}, "State Subsystems":cluster{"PA":bool, "MA":bool, "ns FE":bool, "fs FE":bool, "PA ED":bool, "In.-Box":bool, "MAS":bool, "Booster":bool, "Mirrortower":bool, "Compressor":bool, "Experiment LB":bool, "Experiment LL":bool, "uOPA":bool}, "Status Subscriber Information":T23, "Refs BL uOPA":refnum<vi>[], "PA_Input_2_Beam_6PWpGUI not linked?":bool, "PA_Input_Delay_6PGUI not linked?":bool, "Settings":T26}
  T23 = typedef "PH_Beamline.lvlib/PH_Beamline.Status Subscriber Information.ctl" = cluster{"fs Swich YLF":T24, "fs Exit Shutter":T24, "ns Exit Shutter":T24, "PA Input Shutter":T24, "PA PC WP":T24, "PA PC WP 2":T24, "PA Bypass In":T24, "PA Bypass Out":T24, "PA CH 1":T24, "PA delayed":T24, "PA non delayed":T24, "PA Exit Shutter":T24, "PA Switch Lab":T24, "PA Bridge CH Input MA":T24, "MA Diffusor IB":T24, "MA IB Ready":T24, "MA CH 1":T24, "MA CH 2":T24, "MA CH 3":T24, "MA CH 4":T24, "MA Shutter Align Cam":T24, "MA Position MM5":T24, "Calorimeter Switch":T24, "BL Z6 CH 9":T24, "BL Z6 Beamdump":T24, "BL Z6 Shutter":T24, "COS Sensitivity Switch":T24, "Exp LB Shutter":T24, "Exp LB TB 2":T24, "Exp LB TB 3":T24, "PA LL Input CH":T24, "PA LL Output CH":T24, "LL Comp Input Shutter":T24, "LL Comp Output Shutter":T24, "LL Comp FF Shutter":T24, "Exp LL Shutter":T24, "MA IM In IB":T24, "MA IM Out IB":T24, "MA DB In IB":T24, "MA DB Out IB":T24, "Exp LB Shutter Interlock":T24, "Exp LL Shutter Interlock":T24, "MM1 Force Sensor":T24}
  T24 = typedef "PH_BL-Master.lvlib/PH_BL-Master.Status Subscriber Information.ctl" = cluster{"Index of element":i32, "Attributeset":T25}
  T25 = typedef "PH_BL-Master.lvlib/PH_BL-Master.Attribute Set.ctl" = enum16{"Boolean Status Service Subscriber", "Picture Status Service Subscriber"}
  T26 = typedef "PH_Beamline_Chief.lvlib/PH_Beamline_Chief.Settings.ctl" = cluster{"PA Doublepass Mode":bool, "Compressor Vaccuum LB not relevant":bool, "Windowshutter TB2 not relevant":bool, "Windowshutter TB3 not relevant":bool}
  T27 = typedef "PH_StatusHandler.lvlib/PH_StatusHandler.Status.ctl" = i16
  T28 = typedef "PH_BL-Master.lvlib/PH_BL-Master.i attribute.ctl" = cluster{"Remote controlled":bool, "Boolean Condition Service Subscriber":refnum<vi>[], "Picture Condition Service Subscriber":refnum<vi>[], "R2S":cluster{"GUI Ref":refnum<vi>, "State":bool}, "Vacua":cluster{"GUI Ref":refnum<vi>, "Limit":dbl, "Curr Value":dbl, "in range":bool}[], "O2 Inspection":cluster{"GUI Ref":refnum<vi>, "Concentration":dbl, "State":T27}[], "Boolean Status Service Subscriber":cluster{"GUI Ref":refnum<vi>, "Status":T27, "no Link?":bool, "Status Subscriber Class":T29}[], "Picture Status Service Subscriber":cluster{"GUI Ref":refnum<vi>, "Status":T27, "no Link?":bool, "Status Subscriber Class":T29}[], "6P 4Q Service Subscriber":cluster{"GUI Ref":refnum<vi>, "Selector":T30, "no Link?":bool}[], "Index of latest 6P 4Q changing Instance":i32, "Index of latest Picture Status changing Instance":i32, "Index of latest Boolean Status changing Instance":i32, "Vision ID on same Node":string, "Start Phase over?":bool, "GUI Ref Delete":refnum<vi>}
  T29 = typedef "PH_BL-Master.lvlib/PH_BL-Master.Status Subscriber Class.ctl" = enum16{"unknown", "Switch", "BB", "6P Switch", "Switch GUI", "Switch and 6P State", "Force Sensor"}
  T30 = typedef "PH_4_Pos_Selector.lvlib/PH_4_Pos_Selector.Position Selector.ctl" = u16
  T31 = enum16{"PCS", "Laser", "Vision", "PP", "Special", "Beckhoff"}
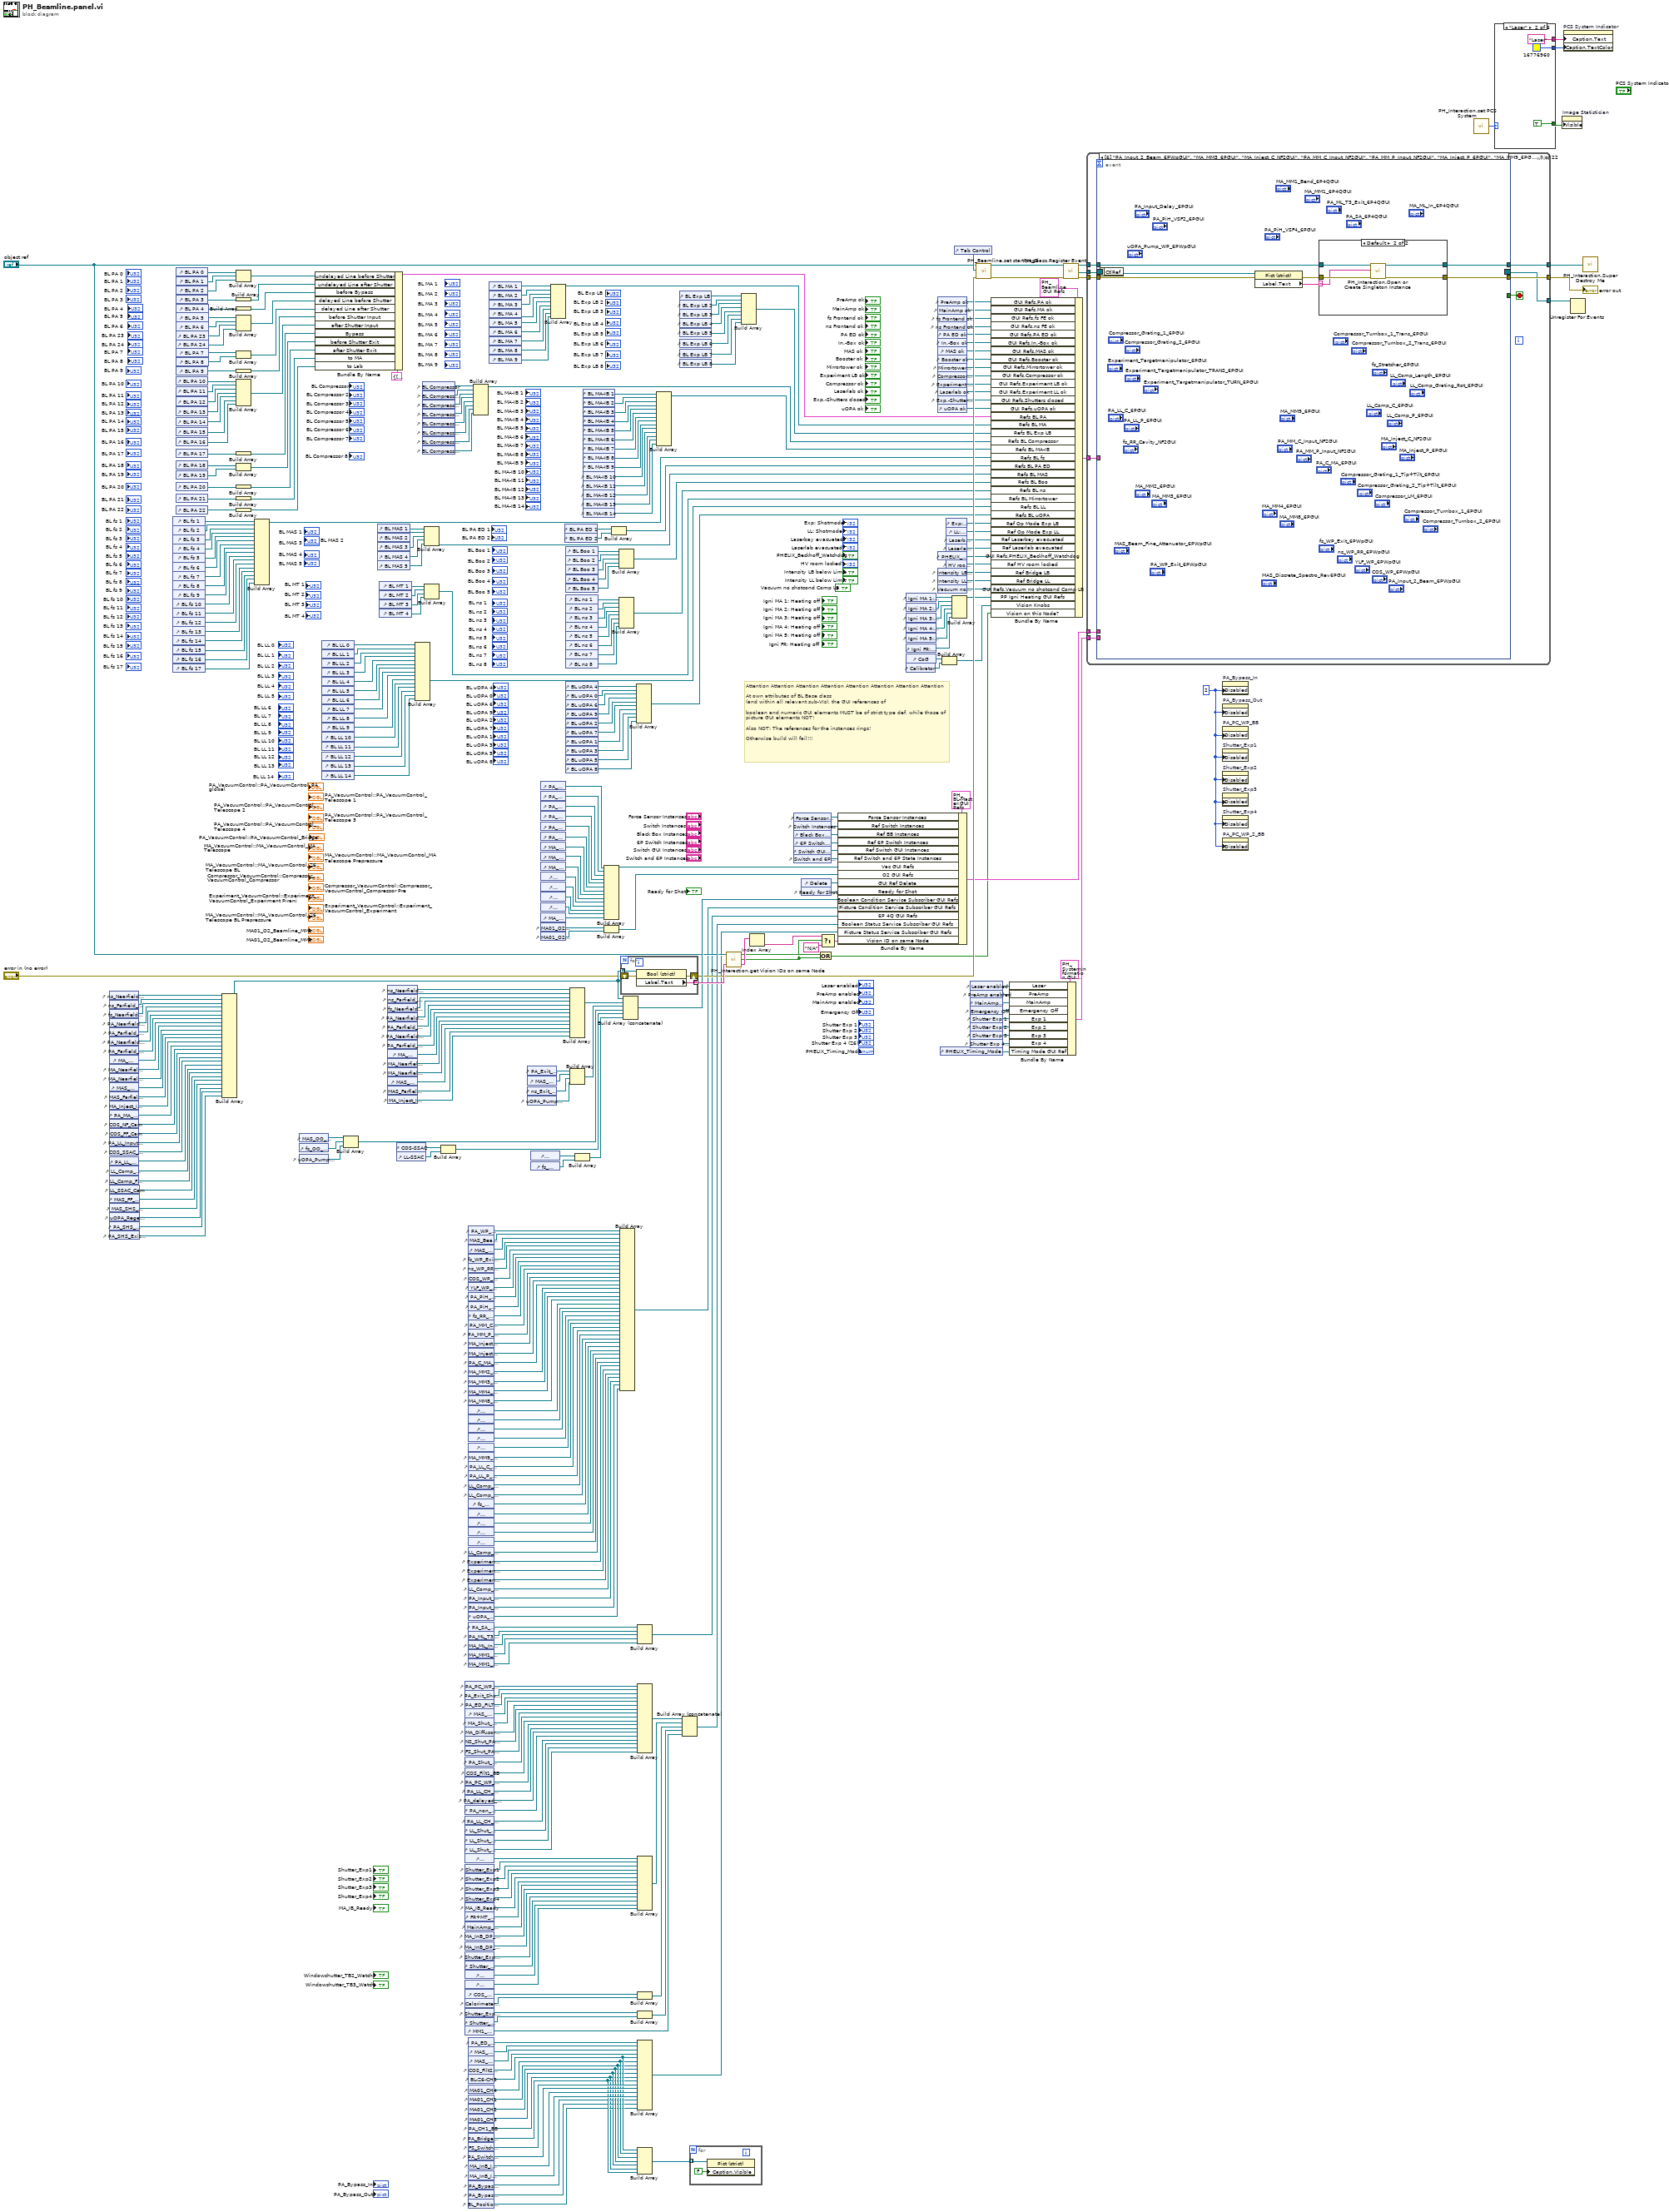
[diagram p0: block diagram]
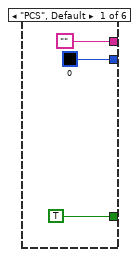
[diagram p2: hidden frame]
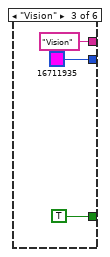
[diagram p3: hidden frame]
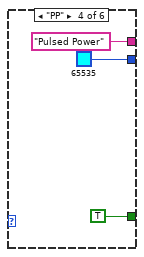
[diagram p4: hidden frame]
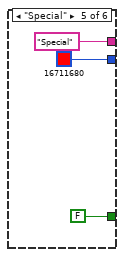
[diagram p5: hidden frame]
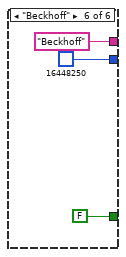
[diagram p6: hidden frame]
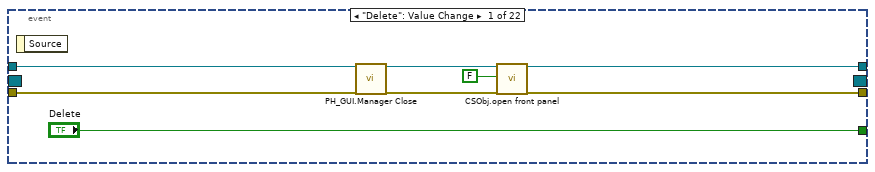
[diagram p7: hidden frame]
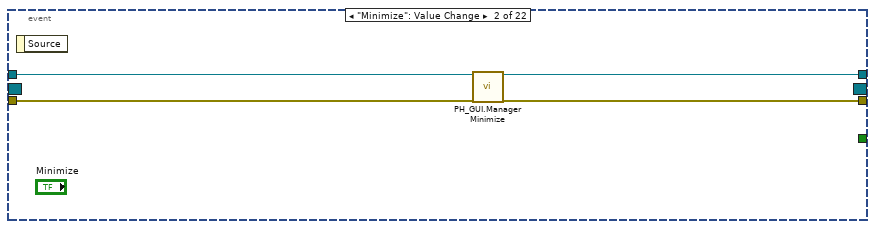
[diagram p8: hidden frame]
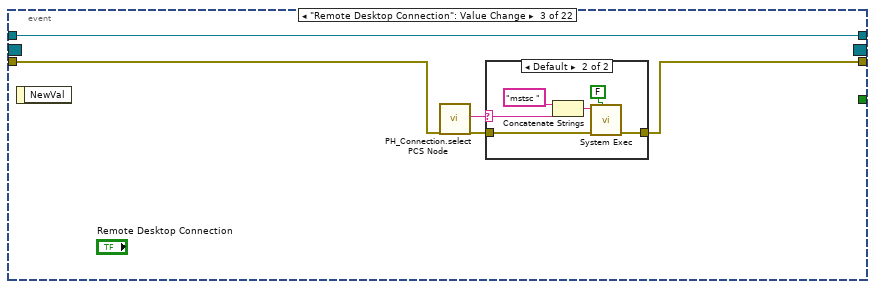
[diagram p9: hidden frame]
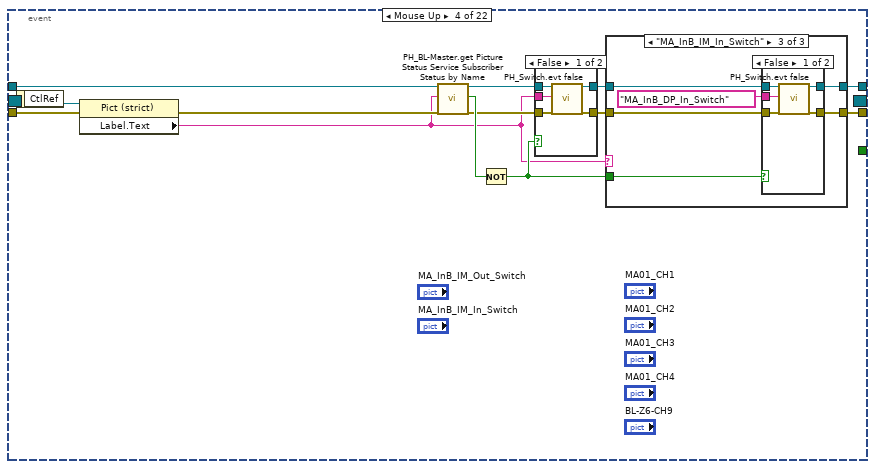
[diagram p11: hidden frame]
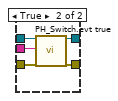
[diagram p12: hidden frame]
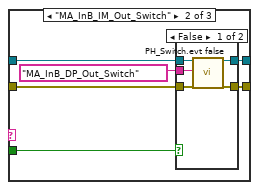
[diagram p14: hidden frame]
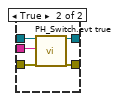
[diagram p15: hidden frame]
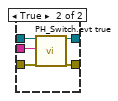
[diagram p16: hidden frame]
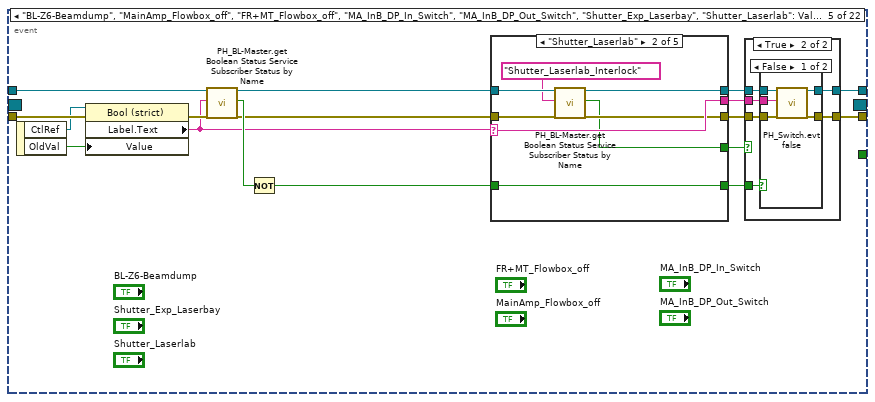
[diagram p17: hidden frame]
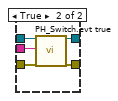
[diagram p19: hidden frame]
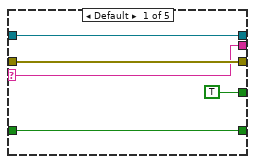
[diagram p20: hidden frame]
diagram:
  w258 = u8 2 ("Disabled")
  # "Attention Attention Attention Attention Attention Attention Attention Attention\n\nAt own attributes of BL Base class \n(and within all relevant sub-VIs), the GUI references of\n\nboolean and numeric GUI elements MUST be of strict type def, while those of\npicture GUI elements NOT!\n\nAlso NOT: The references for the instances rings!\n\nOtherwise build will fail!!!"
  n1 = control-ref of="ns_Nearfield_Ring_Exit_Cam"() -> (w416:refnum<vi>)
  n2 = control-ref of="ns_Farfield_Ring_Exit_Cam"() -> (w415:refnum<vi>)
  n3 = control-ref of="fs_Nearfield_Frontend_Cam"() -> (w414:refnum<vi>)
  n4 = control-ref of="PA_Nearfield_Input_Cam"() -> (w413:refnum<vi>)
  n5 = control-ref of="PA_Farfield_Input_Cam"() -> (w412:refnum<vi>)
  n6 = control-ref of="PA_Nearfield_Exit_Cam"() -> (w411:refnum<vi>)
  n7 = control-ref of="PA_Farfield_Exit_Cam"() -> (w410:refnum<vi>)
  n8 = control-ref of="MA_Alignment_Cam"() -> (w409:refnum<vi>)
  n9 = control-ref of="MA_Nearfield_PiH_in_Cam"() -> (w408:refnum<vi>)
  n10 = control-ref of="MA_Nearfield_PiH_out_Cam"() -> (w407:refnum<vi>)
  n11 = control-ref of="MAS_Nearfield_Cam"() -> (w406:refnum<vi>)
  n12 = control-ref of="MAS_Farfield_High_Res_Cam"() -> (w405:refnum<vi>)
  n13 = control-ref of="MA_Inject_In_Cam"() -> (w354:refnum<vi>)
  n14 = control-ref of="PA_MA_Bridge_Input_Cam"() -> (w322:refnum<vi>)
  n15 = control-ref of="COS_NF_Cam"() -> (w288:refnum<vi>)
  n16 = control-ref of="COS_FF_Cam"() -> (w287:refnum<vi>)
  n17 = control-ref of="PA_LL_Input_Cam"() -> (w255:refnum<vi>)
  n18 = control-ref of="COS_SSAC_Cam"() -> (w211:refnum<vi>)
  n19 = control-ref of="PA_LL_Output_Cam"() -> (w151:refnum<vi>)
  n20 = control-ref of="LL_Comp_Input_Cam"() -> (w150:refnum<vi>)
  n21 = control-ref of="LL_Comp_FF_Cam"() -> (w149:refnum<vi>)
  n22 = control-ref of="LL_SSAC_Cam"() -> (w144:refnum<vi>)
  n23 = control-ref of="MAS_FF_HamamatsuCam"() -> (w96:refnum<vi>)
  n24 = control-ref of="MAS_SHS_Cam"() -> (w95:refnum<vi>)
  n25 = control-ref of="uOPA_Regen_Cam"() -> (w84:refnum<vi>)
  n26 = control-ref of="PA_SHS_Input_Cam"() -> (w19:refnum<vi>)
  n27 = control-ref of="PA_SHS_Exit_Cam"() -> (w18:refnum<vi>)
  n28 = control-ref of="BL fs 1"() -> (w381:refnum<vi>)
  n29 = control-ref of="BL fs 2"() -> (w380:refnum<vi>)
  n30 = control-ref of="BL fs 3"() -> (w379:refnum<vi>)
  n31 = control-ref of="BL fs 4"() -> (w378:refnum<vi>)
  n32 = control-ref of="BL fs 5"() -> (w377:refnum<vi>)
  n33 = control-ref of="BL fs 6"() -> (w376:refnum<vi>)
  n34 = control-ref of="BL fs 7"() -> (w375:refnum<vi>)
  n35 = control-ref of="BL fs 8"() -> (w374:refnum<vi>)
  n36 = control-ref of="BL fs 9"() -> (w373:refnum<vi>)
  n37 = control-ref of="BL fs 10"() -> (w372:refnum<vi>)
  n38 = control-ref of="BL fs 11"() -> (w371:refnum<vi>)
  n39 = control-ref of="BL fs 12"() -> (w370:refnum<vi>)
  n40 = control-ref of="BL fs 13"() -> (w369:refnum<vi>)
  n41 = control-ref of="BL fs 14"() -> (w323:refnum<vi>)
  n42 = control-ref of="BL fs 15"() -> (w282:refnum<vi>)
  n43 = control-ref of="BL fs 16"() -> (w281:refnum<vi>)
  n44 = control-ref of="BL fs 17"() -> (w280:refnum<vi>)
  n45 = control-ref of="BL PA 0"() -> (w248:refnum<vi>)
  n46 = control-ref of="BL PA 1"() -> (w247:refnum<vi>)
  n47 = control-ref of="BL PA 2"() -> (w246:refnum<vi>)
  n48 = control-ref of="BL PA 3"() -> (w244:refnum<vi>)
  n49 = control-ref of="BL PA 9"() -> (w234:refnum<vi>)
  n50 = control-ref of="BL PA 10"() -> (w232:refnum<vi>)
  n51 = control-ref of="BL PA 11"() -> (w231:refnum<vi>)
  n52 = control-ref of="BL PA 12"() -> (w230:refnum<vi>)
  n53 = control-ref of="BL PA 13"() -> (w229:refnum<vi>)
  n54 = control-ref of="BL PA 14"() -> (w228:refnum<vi>)
  n55 = control-ref of="BL PA 15"() -> (w227:refnum<vi>)
  n56 = control-ref of="BL PA 16"() -> (w226:refnum<vi>)
  n57 = control-ref of="BL PA 17"() -> (w224:refnum<vi>)
  n58 = control-ref of="BL PA 18"() -> (w222:refnum<vi>)
  n59 = control-ref of="BL PA 19"() -> (w221:refnum<vi>)
  n60 = control-ref of="BL PA 20"() -> (w219:refnum<vi>)
  n61 = control-ref of="BL PA 21"() -> (w218:refnum<vi>)
  n62 = control-ref of="BL PA 22"() -> (w217:refnum<vi>)
  n63 = control-ref of="BL PA 4"() -> (w242:refnum<vi>)
  n64 = control-ref of="BL PA 5"() -> (w240:refnum<vi>)
  n65 = control-ref of="BL PA 6"() -> (w239:refnum<vi>)
  n66 = control-ref of="BL PA 23"() -> (w21:refnum<vi>)
  n67 = control-ref of="BL PA 24"() -> (w20:refnum<vi>)
  n68 = control-ref of="BL PA 7"() -> (w237:refnum<vi>)
  n69 = control-ref of="BL PA 8"() -> (w236:refnum<vi>)
  n70 = Build Array(w416, w415, w414, w413, w412, w411, w410, w409, w408, w407, w406, w405, w354, w322, w288, w287, w255, w211, w151, w150, w149, w144, w96, w95, w84, w19, w18) -> (w108:refnum<vi>[])
  n71 = Build Array(w248, w247, w246) -> (w245:refnum<vi>[])
  n72 = Build Array(w244) -> (w243:refnum<vi>[])
  n73 = Build Array(w242) -> (w241:refnum<vi>[])
  n74 = Build Array(w240, w239, w21, w20) -> (w238:refnum<vi>[])
  n75 = Build Array(w237, w236) -> (w235:refnum<vi>[])
  n76 = Build Array(w234) -> (w233:refnum<vi>[])
  n77 = Build Array(w232, w231, w230, w229, w228, w227, w226) -> (w225:refnum<vi>[])
  n78 = Build Array(w224) -> (w223:refnum<vi>[])
  n79 = Build Array(w222, w221) -> (w220:refnum<vi>[])
  n80 = Build Array(w219) -> (w216:refnum<vi>[])
  n81 = Build Array(w218) -> (w215:refnum<vi>[])
  n82 = Build Array(w217) -> (w214:refnum<vi>[])
  n83 = Build Array(w381, w380, w379, w378, w377, w376, w375, w374, w373, w372, w371, w370, w369, w323, w282, w281, w280) -> (w43:refnum<vi>[])
  n84 = control-ref of="MAS_OO_Spectrometer"() -> (w270:refnum<vi>)
  n85 = control-ref of="fs_OO_Spectrometer"() -> (w269:refnum<vi>)
  n86 = control-ref of="uOPA_Pump_OO_Spectrometer"() -> (w83:refnum<vi>)
  n87 = Bundle By Name(cluster=T19 {"undelayed Line before Shutter"=[], "undelayed Line after Shutter"=[], "before Bypass"=[], "delayed Line before Shutter"=[], "delayed Line after Shutter"=[], "before Shutter Input"=[], "after Shutter Input"=[], "Bypass"=[], "before Shutter Exit"=[], "after Shutter Exit"=[], "to MA"=[], "to Lab"=[]} ("Refs BL PA"), "undelayed Line before Shutter"=w245, "undelayed Line after Shutter"=w243, "before Bypass"=w241, "delayed Line before Shutter"=w238, "delayed Line after Shutter"=w235, "before Shutter Input"=w233, "after Shutter Input"=w225, "Bypass"=w223, "before Shutter Exit"=w220, "after Shutter Exit"=w216, "to MA"=w215, "to Lab"=w214) -> (w38:T19)
  n88 = control-ref of="BL LL 0"() -> (w274:refnum<vi>)
  n89 = control-ref of="BL LL 1"() -> (w273:refnum<vi>)
  n90 = control-ref of="BL LL 2"() -> (w254:refnum<vi>)
  n91 = control-ref of="BL LL 3"() -> (w253:refnum<vi>)
  n92 = control-ref of="BL LL 4"() -> (w252:refnum<vi>)
  n93 = control-ref of="BL LL 5"() -> (w250:refnum<vi>)
  n94 = control-ref of="BL LL 6"() -> (w161:refnum<vi>)
  n95 = control-ref of="BL LL 7"() -> (w160:refnum<vi>)
  n96 = control-ref of="BL LL 8"() -> (w159:refnum<vi>)
  n97 = control-ref of="BL LL 9"() -> (w158:refnum<vi>)
  n98 = control-ref of="BL LL 10"() -> (w157:refnum<vi>)
  n99 = control-ref of="BL LL 11"() -> (w156:refnum<vi>)
  n100 = control-ref of="BL LL 12"() -> (w155:refnum<vi>)
  n101 = control-ref of="BL LL 13"() -> (w154:refnum<vi>)
  n102 = control-ref of="BL LL 14"() -> (w142:refnum<vi>)
  n103 = Build Array(w270, w269, w83) -> (w119:refnum<vi>[])
  n104 = control-ref of="BL MAS 1"() -> (w362:refnum<vi>)
  n105 = control-ref of="BL MAS 2"() -> (w361:refnum<vi>)
  n106 = control-ref of="BL MAS 3"() -> (w97:refnum<vi>)
  n107 = control-ref of="BL MAS 4"() -> (w360:refnum<vi>)
  n108 = control-ref of="BL MAS 5"() -> (w359:refnum<vi>)
  n109 = control-ref of="BL MT 1"() -> (w339:refnum<vi>)
  n110 = control-ref of="BL MT 2"() -> (w338:refnum<vi>)
  n111 = control-ref of="BL MT 3"() -> (w337:refnum<vi>)
  n112 = control-ref of="BL MT 4"() -> (w332:refnum<vi>)
  n113 = control-ref of="ns_Nearfield_Ring_Exit_ImageOperator"() -> (w404:refnum<vi>)
  n114 = control-ref of="ns_Farfield_Ring_Exit_ImageOperator"() -> (w403:refnum<vi>)
  n115 = control-ref of="fs_Nearfield_Frontend_ImageOperator"() -> (w402:refnum<vi>)
  n116 = control-ref of="PA_Nearfield_Input_ImageOperator"() -> (w401:refnum<vi>)
  n117 = control-ref of="PA_Farfield_Input_ImageOperator"() -> (w400:refnum<vi>)
  n118 = control-ref of="PA_Nearfield_Exit_ImageOperator"() -> (w399:refnum<vi>)
  n119 = control-ref of="PA_Farfield_Exit_ImageOperator"() -> (w398:refnum<vi>)
  n120 = control-ref of="MA_Alignment_ImageOperator"() -> (w397:refnum<vi>)
  n121 = control-ref of="MA_Nearfield_PiH_in_ImageOperator"() -> (w396:refnum<vi>)
  n122 = control-ref of="MA_Nearfield_PiH_out_ImageOperator"() -> (w395:refnum<vi>)
  n123 = control-ref of="MAS_Nearfield_ImageOperator"() -> (w394:refnum<vi>)
  n124 = control-ref of="MAS_Farfield_High_Res_ImageOperator"() -> (w393:refnum<vi>)
  n125 = control-ref of="MA_Inject_In_ImageOperator"() -> (w355:refnum<vi>)
  n126 = control-ref of="COS-SSAC"() -> (w210:refnum<vi>)
  n127 = control-ref of="LL-SSAC"() -> (w143:refnum<vi>)
  n128 = Build Array(w274, w273, w254, w253, w252, w250, w161, w160, w159, w158, w157, w156, w155, w154, w142) -> (w49:refnum<vi>[])
  n129 = control-ref of="BL Compressor"() -> (w304:refnum<vi>)
  n130 = control-ref of="BL Compressor 2"() -> (w303:refnum<vi>)
  n131 = control-ref of="BL Compressor 3"() -> (w302:refnum<vi>)
  n132 = control-ref of="BL Compressor 4"() -> (w301:refnum<vi>)
  n133 = control-ref of="BL Compressor 5"() -> (w300:refnum<vi>)
  n134 = control-ref of="BL Compressor 6"() -> (w299:refnum<vi>)
  n135 = control-ref of="BL Compressor 7"() -> (w298:refnum<vi>)
  n136 = control-ref of="BL Compressor 8"() -> (w279:refnum<vi>)
  n137 = Build Array(w362, w361, w97, w360, w359) -> (w45:refnum<vi>[])
  n138 = Build Array(w339, w338, w337, w332) -> (w48:refnum<vi>[])
  n139 = Build Array(w210, w143) -> (w118:refnum<vi>[])
  n140 = control-ref of="PA_PC_WP_BB"() -> (w383:refnum<vi>)
  n141 = control-ref of="PA_Exit_Shut_BB"() -> (w382:refnum<vi>)
  n142 = control-ref of="PA_ED_FILT1_BB"() -> (w366:refnum<vi>)
  n143 = control-ref of="MAS_Attenuator_1_BB"() -> (w365:refnum<vi>)
  n144 = control-ref of="MA_Shut_AlignCam_BB"() -> (w356:refnum<vi>)
  n145 = control-ref of="MA_Diffusor_Inject_In_BB"() -> (w195:refnum<vi>)
  n146 = control-ref of="NS_Shut_PA_BB"() -> (w328:refnum<vi>)
  n147 = control-ref of="FS_Shut_PA_BB"() -> (w325:refnum<vi>)
  n148 = control-ref of="PA_Shut_Input_BB"() -> (w324:refnum<vi>)
  n149 = control-ref of="COS_Filt1_BB"() -> (w289:refnum<vi>)
  n150 = control-ref of="PA_PC_WP_2_BB"() -> (w260:refnum<vi>)
  n151 = control-ref of="PA_LL_CH_Input_BB"() -> (w251:refnum<vi>)
  n152 = control-ref of="PA_delayed_BB"() -> (w213:refnum<vi>)
  n153 = control-ref of="PA_non_delayed_BB"() -> (w212:refnum<vi>)
  n154 = control-ref of="PA_LL_CH_Output_BB"() -> (w148:refnum<vi>)
  n155 = control-ref of="LL_Shut_Comp_Input_BB"() -> (w147:refnum<vi>)
  n156 = control-ref of="LL_Shut_Comp_FF_BB"() -> (w146:refnum<vi>)
  n157 = control-ref of="LL_Shut_Comp_Output_BB"() -> (w145:refnum<vi>)
  n158 = control-ref of="BL-Z6-Beamdump"() -> (w340:refnum<vi>)
  n159 = control-ref of="Shutter_Exp1"() -> (w336:refnum<vi>)
  n160 = control-ref of="Shutter_Exp2"() -> (w335:refnum<vi>)
  n161 = control-ref of="Shutter_Exp3"() -> (w334:refnum<vi>)
  n162 = control-ref of="Shutter_Exp4"() -> (w333:refnum<vi>)
  n163 = control-ref of="MA_IB_Ready"() -> (w331:refnum<vi>)
  n164 = control-ref of="FR+MT_Flowbox_off"() -> (w330:refnum<vi>)
  n165 = control-ref of="MainAmp_Flowbox_off"() -> (w329:refnum<vi>)
  n166 = control-ref of="MA_InB_DP_In_Switch"() -> (w306:refnum<vi>)
  n167 = control-ref of="MA_InB_DP_Out_Switch"() -> (w305:refnum<vi>)
  n168 = control-ref of="Shutter_Exp_Laserbay"() -> (w276:refnum<vi>)
  n169 = control-ref of="Shutter_Laserlab"() -> (w275:refnum<vi>)
  n170 = control-ref of="Windowshutter_TB2_Watch"() -> (w259:refnum<vi>)
  n171 = control-ref of="Windowshutter_TB3_Watch"() -> (w199:refnum<vi>)
  n172 = control-ref of="COS_Sensitivity_Switch"() -> (w286:refnum<vi>)
  n173 = control-ref of="Calorimeter_Switch"() -> (w284:refnum<vi>)
  n174 = control-ref of="Shutter_Exp_Laserbay_Interlock"() -> (w272:refnum<vi>)
  n175 = control-ref of="Shutter_Laserlab_Interlock"() -> (w271:refnum<vi>)
  n176 = control-ref of="MM1_ForceSensor"() -> (w15:refnum<vi>)
  n177 = control-ref of="PA_WP_Exit_6PWpGUI"() -> (w192:refnum<vi>)
  n178 = control-ref of="MAS_Beam_Fine_Attenuator_6PWpGUI"() -> (w191:refnum<vi>)
  n179 = control-ref of="MAS_Discrete_Spectro_6PGUI"() -> (w190:refnum<vi>)
  n180 = control-ref of="fs_WP_Exit_6PWpGUI"() -> (w189:refnum<vi>)
  n181 = control-ref of="ns_WP_RR_6PWpGUI"() -> (w188:refnum<vi>)
  n182 = control-ref of="COS_WP_6PWpGUI"() -> (w187:refnum<vi>)
  n183 = control-ref of="YLF_WP_6PWpGUI"() -> (w186:refnum<vi>)
  n184 = control-ref of="PA_PiH_VSF2_6PGUI"() -> (w185:refnum<vi>)
  n185 = control-ref of="PA_PiH_VSF4_6PGUI"() -> (w184:refnum<vi>)
  n186 = control-ref of="fs_RR_Cavity_NF2GUI"() -> (w179:refnum<vi>)
  n187 = control-ref of="PA_MM_C_Input_NF2GUI"() -> (w178:refnum<vi>)
  n188 = control-ref of="PA_MM_P_Input_NF2GUI"() -> (w177:refnum<vi>)
  n189 = control-ref of="MA_Inject_C_NF2GUI"() -> (w176:refnum<vi>)
  n190 = control-ref of="MA_Inject_P_6PGUI"() -> (w175:refnum<vi>)
  n191 = control-ref of="PA_C_MA_6PGUI"() -> (w174:refnum<vi>)
  n192 = control-ref of="MA_MM2_6PGUI"() -> (w173:refnum<vi>)
  n193 = control-ref of="MA_MM3_6PGUI"() -> (w172:refnum<vi>)
  n194 = control-ref of="MA_MM4_6PGUI"() -> (w171:refnum<vi>)
  n195 = control-ref of="MA_MM8_6PGUI"() -> (w170:refnum<vi>)
  n196 = control-ref of="Compressor_Grating_1_Tip+Tilt_6PGUI"() -> (w169:refnum<vi>)
  n197 = control-ref of="Compressor_Grating_2_Tip+Tilt_6PGUI"() -> (w168:refnum<vi>)
  n198 = control-ref of="Compressor_LM_6PGUI"() -> (w167:refnum<vi>)
  n199 = control-ref of="Compressor_Turnbox_1_6PGUI"() -> (w166:refnum<vi>)
  n200 = control-ref of="Compressor_Turnbox_2_6PGUI"() -> (w165:refnum<vi>)
  n201 = control-ref of="MA_MM9_6PGUI"() -> (w164:refnum<vi>)
  n202 = control-ref of="PA_LL_C_6PGUI"() -> (w163:refnum<vi>)
  n203 = control-ref of="PA_LL_P_6PGUI"() -> (w162:refnum<vi>)
  n204 = control-ref of="LL_Comp_C_6PGUI"() -> (w153:refnum<vi>)
  n205 = control-ref of="LL_Comp_P_6PGUI"() -> (w152:refnum<vi>)
  n206 = control-ref of="fs_Stretcher_6PGUI"() -> (w141:refnum<vi>)
  n207 = control-ref of="Compressor_Grating_1_6PGUI"() -> (w140:refnum<vi>)
  n208 = control-ref of="Compressor_Grating_2_6PGUI"() -> (w139:refnum<vi>)
  n209 = control-ref of="Compressor_Turnbox_1_Trans_6PGUI"() -> (w138:refnum<vi>)
  n210 = control-ref of="Compressor_Turnbox_2_Trans_6PGUI"() -> (w137:refnum<vi>)
  n211 = control-ref of="LL_Comp_Length_6PGUI"() -> (w136:refnum<vi>)
  n212 = control-ref of="Experiment_Targetmanipulator_TRANS_6PGUI"() -> (w135:refnum<vi>)
  n213 = control-ref of="Experiment_Targetmanipulator_6PGUI"() -> (w134:refnum<vi>)
  n214 = control-ref of="Experiment_Targetmanipulator_TURN_6PGUI"() -> (w133:refnum<vi>)
  n215 = control-ref of="LL_Comp_Grating_Rot_6PGUI"() -> (w132:refnum<vi>)
  n216 = control-ref of="PA_Input_Delay_6PGUI"() -> (w131:refnum<vi>)
  n217 = control-ref of="PA_Input_2_Beam_6PWpGUI"() -> (w102:refnum<vi>)
  n218 = control-ref of="uOPA_Pump_WP_6PWpGUI"() -> (w81:refnum<vi>)
  n219 = control-ref of="PA_SA_6P4QGUI"() -> (w112:refnum<vi>)
  n220 = control-ref of="PA_ML_T3_Exit_6P4QGUI"() -> (w111:refnum<vi>)
  n221 = control-ref of="MA_ML_In_6P4QGUI"() -> (w101:refnum<vi>)
  n222 = control-ref of="MA_MM1_6P4QGUI"() -> (w17:refnum<vi>)
  n223 = control-ref of="MA_MM1_Bend_6P4QGUI"() -> (w16:refnum<vi>)
  n224 = control-ref of="PA_ED_FILT2_BB"() -> (w194:refnum<vi>)
  n225 = control-ref of="MAS_Attenuator_2_BB"() -> (w99:refnum<vi>)
  n226 = control-ref of="MAS_Attenuator_3_BB"() -> (w98:refnum<vi>)
  n227 = control-ref of="COS_Filt2_BB"() -> (w193:refnum<vi>)
  n228 = control-ref of="BL-Z6-CH9"() -> (w129:refnum<vi>)
  n229 = control-ref of="MA01_CH4"() -> (w128:refnum<vi>)
  n230 = control-ref of="MA01_CH1"() -> (w127:refnum<vi>)
  n231 = control-ref of="MA01_CH2"() -> (w126:refnum<vi>)
  n232 = control-ref of="MA01_CH3"() -> (w125:refnum<vi>)
  n233 = control-ref of="PA_CH1_BB"() -> (w109:refnum<vi>)
  n234 = control-ref of="PA_Bridge_CH_Input_MA_BB"() -> (w124:refnum<vi>)
  n235 = control-ref of="FS_Switch_YLF_BB"() -> (w183:refnum<vi>)
  n236 = control-ref of="PA_Switch_Lab_BB"() -> (w182:refnum<vi>)
  n237 = control-ref of="MA_InB_IM_Out_Switch"() -> (w181:refnum<vi>)
  n238 = control-ref of="MA_InB_IM_In_Switch"() -> (w180:refnum<vi>)
  n239 = control-ref of="PA_Bypass_In"() -> (w123:refnum<vi>)
  n240 = control-ref of="PA_Bypass_Out"() -> (w122:refnum<vi>)
  n241 = control-ref of="BL_Position_MM5::MA_MM5_6PGUI"() -> (w110:refnum<vi>)
  n242 = Build Array(w304, w303, w302, w301, w300, w299, w298, w279) -> (w41:refnum<vi>[])
  n243 = control-ref of="BL MA 1"() -> (w424:refnum<vi>)
  n244 = control-ref of="BL MA 2"() -> (w423:refnum<vi>)
  n245 = control-ref of="BL MA 3"() -> (w422:refnum<vi>)
  n246 = control-ref of="BL MA 4"() -> (w421:refnum<vi>)
  n247 = control-ref of="BL MA 5"() -> (w417:refnum<vi>)
  n248 = control-ref of="BL MA 6"() -> (w420:refnum<vi>)
  n249 = control-ref of="BL MA 7"() -> (w419:refnum<vi>)
  n250 = control-ref of="BL MA 8"() -> (w418:refnum<vi>)
  n251 = control-ref of="BL MA 9"() -> (w320:refnum<vi>)
  n252 = control-ref of="PA_Exit_Powermeter"() -> (w364:refnum<vi>)
  n253 = control-ref of="MAS_Powermeter"() -> (w363:refnum<vi>)
  n254 = control-ref of="ns_Exit_Powermeter"() -> (w349:refnum<vi>)
  n255 = control-ref of="uOPA_Pump_Powermeter"() -> (w82:refnum<vi>)
  n256 = control-ref of="PA-Backreflection-Meas"() -> (w261:refnum<vi>)
  n257 = control-ref of="fs_Synchrolock_Watch"() -> (w200:refnum<vi>)
  n258 = control-ref of="PA_VacuumControl::PA_VacuumControl_PA global"() -> (w392:refnum<vi>)
  n259 = control-ref of="PA_VacuumControl::PA_VacuumControl_Telescope 1"() -> (w391:refnum<vi>)
  n260 = control-ref of="PA_VacuumControl::PA_VacuumControl_Telescope 2"() -> (w390:refnum<vi>)
  n261 = control-ref of="PA_VacuumControl::PA_VacuumControl_Telescope 3"() -> (w389:refnum<vi>)
  n262 = control-ref of="PA_VacuumControl::PA_VacuumControl_Telescope 4"() -> (w388:refnum<vi>)
  n263 = control-ref of="PA_VacuumControl::PA_VacuumControl_Bridge"() -> (w387:refnum<vi>)
  n264 = control-ref of="MA_VacuumControl::MA_VacuumControl_MA Telescope"() -> (w386:refnum<vi>)
  n265 = control-ref of="MA_VacuumControl::MA_VacuumControl_MA Telescope Prepressure"() -> (w385:refnum<vi>)
  n266 = control-ref of="MA_VacuumControl::MA_VacuumControl_Z6 Telescope BL"() -> (w321:refnum<vi>)
  n267 = control-ref of="Compressor_VacuumControl::Compressor_VacuumControl_Compressor"() -> (w294:refnum<vi>)
  n268 = control-ref of="Compressor_VacuumControl::Compressor_VacuumControl_Compressor Pre"() -> (w293:refnum<vi>)
  n269 = control-ref of="Experiment_VacuumControl::Experiment_VacuumControl_Experiment Pirani"() -> (w257:refnum<vi>)
  n270 = control-ref of="Experiment_VacuumControl::Experiment_VacuumControl_Experiment"() -> (w256:refnum<vi>)
  n271 = control-ref of="MA_VacuumControl::MA_VacuumControl_Z6 Telescope BL Prepressure"() -> (w100:refnum<vi>)
  n272 = control-ref of="MA01_O2_Beamline_MM1"() -> (w358:refnum<vi>)
  n273 = control-ref of="MA01_O2_Beamline_MM3"() -> (w357:refnum<vi>)
  n274 = Build Array(w424, w423, w422, w421, w417, w420, w419, w418, w320) -> (w39:refnum<vi>[])
  n275 = control-ref of="BL PA ED 1"() -> (w368:refnum<vi>)
  n276 = control-ref of="BL PA ED 2"() -> (w367:refnum<vi>)
  n277 = control-ref of="BL Boo 1"() -> (w353:refnum<vi>)
  n278 = control-ref of="BL Boo 2"() -> (w352:refnum<vi>)
  n279 = control-ref of="BL Boo 3"() -> (w351:refnum<vi>)
  n280 = control-ref of="BL Boo 4"() -> (w350:refnum<vi>)
  n281 = control-ref of="BL Boo 5"() -> (w285:refnum<vi>)
  n282 = control-ref of="BL ns 1"() -> (w348:refnum<vi>)
  n283 = control-ref of="BL ns 2"() -> (w347:refnum<vi>)
  n284 = control-ref of="BL ns 3"() -> (w346:refnum<vi>)
  n285 = control-ref of="BL ns 4"() -> (w345:refnum<vi>)
  n286 = control-ref of="BL ns 5"() -> (w344:refnum<vi>)
  n287 = control-ref of="BL ns 6"() -> (w343:refnum<vi>)
  n288 = control-ref of="BL ns 7"() -> (w342:refnum<vi>)
  n289 = control-ref of="BL ns 8"() -> (w341:refnum<vi>)
  n290 = control-ref of="BL uOPA 4"() -> (w94:refnum<vi>)
  n291 = control-ref of="BL uOPA 0"() -> (w93:refnum<vi>)
  n292 = control-ref of="BL uOPA 6"() -> (w92:refnum<vi>)
  n293 = control-ref of="BL uOPA 9"() -> (w91:refnum<vi>)
  n294 = control-ref of="BL uOPA 2"() -> (w90:refnum<vi>)
  n295 = control-ref of="BL uOPA 7"() -> (w89:refnum<vi>)
  n296 = control-ref of="BL uOPA 1"() -> (w88:refnum<vi>)
  n297 = control-ref of="BL uOPA 3"() -> (w87:refnum<vi>)
  n298 = control-ref of="BL uOPA 5"() -> (w86:refnum<vi>)
  n299 = control-ref of="BL uOPA 8"() -> (w85:refnum<vi>)
  n300 = Build Array(w404, w403, w402, w401, w400, w399, w398, w397, w396, w395, w394, w393, w355) -> (w121:refnum<vi>[])
  n301 = Build Array(w364, w363, w349, w82) -> (w120:refnum<vi>[])
  n302 = Build Array(w261, w200) -> (w117:refnum<vi>[])
  n303 = control-ref of="BL MA-IB 1"() -> (w384:refnum<vi>)
  n304 = control-ref of="BL MA-IB 2"() -> (w319:refnum<vi>)
  n305 = control-ref of="BL MA-IB 3"() -> (w318:refnum<vi>)
  n306 = control-ref of="BL MA-IB 4"() -> (w317:refnum<vi>)
  n307 = control-ref of="BL MA-IB 5"() -> (w316:refnum<vi>)
  n308 = control-ref of="BL MA-IB 6"() -> (w315:refnum<vi>)
  n309 = control-ref of="BL MA-IB 7"() -> (w314:refnum<vi>)
  n310 = control-ref of="BL MA-IB 8"() -> (w313:refnum<vi>)
  n311 = control-ref of="BL MA-IB 9"() -> (w312:refnum<vi>)
  n312 = control-ref of="BL MA-IB 10"() -> (w311:refnum<vi>)
  n313 = control-ref of="BL MA-IB 11"() -> (w310:refnum<vi>)
  n314 = control-ref of="BL MA-IB 12"() -> (w309:refnum<vi>)
  n315 = control-ref of="BL MA-IB 13"() -> (w308:refnum<vi>)
  n316 = control-ref of="BL MA-IB 14"() -> (w307:refnum<vi>)
  n317 = Build Array(w392, w391, w390, w389, w388, w387, w386, w385, w321, w294, w293, w257, w256, w100) -> (w74:refnum<vi>[])
  n318 = Build Array(w358, w357) -> (w73:refnum<vi>[])
  n319 = Build Array(w368, w367) -> (w44:refnum<vi>[])
  n320 = Build Array(w353, w352, w351, w350, w285) -> (w46:refnum<vi>[])
  n321 = Build Array(w348, w347, w346, w345, w344, w343, w342, w341) -> (w47:refnum<vi>[])
  n322 = Build Array(w192, w191, w190, w189, w188, w187, w186, w185, w184, w179, w178, w177, w176, w175, w174, w173, w172, w171, w170, w169, w168, w167, w166, w165, w164, w163, w162, w153, w152, w141, w140, w139, w138, w137, w136, w135, w134, w133, w132, w131, w102, w81) -> (w13:refnum<vi>[])
  n323 = for {
    shift-right: [w427] -> w64
    shift-left: "error in (no error)" -> [w428]
    tunnel: w108 -> [w426] mode=indexing
    tunnel: [w425] -> w107 mode=indexing
    n324 = property class="Bool (strict)"(reference=w426, error in=w428) -> (error out=w427:errorcluster, "Label.Text"=w425:string)  [unwired: 1 out]
  }
  n325 = Build Array (concatenate)(w108, w121, w120, w119, w118, w117) -> (w71:refnum<vi>[])
  n326 = Build Array(w94, w93, w92, w91, w90, w89, w88, w87, w86, w85) -> (w50:refnum<vi>[])
  n327 = Build Array(w112, w111, w101, w17, w16) -> (w12:refnum<vi>[])
  n328 = Build Array(w383, w382, w366, w365, w356, w195, w328, w325, w324, w289, w260, w251, w213, w212, w148, w147, w146, w145) -> (w116:refnum<vi>[])
  n329 = Build Array(w340, w336, w335, w334, w333, w331, w330, w329, w306, w305, w276, w275, w259, w199) -> (w115:refnum<vi>[])
  n330 = Build Array(w286, w284) -> (w114:refnum<vi>[])
  n331 = Build Array(w272, w271) -> (w113:refnum<vi>[])
  n332 = Build Array(w194, w99, w98, w193, w129, w128, w127, w126, w125, w109, w124, w183, w182, w181, w180, w123, w122, w110) -> (w6:refnum<vi>[])
  n333 = Build Array(w129, w128, w127, w126, w125, w109, w124) -> (w130:refnum<vi>[])
  n334 = Build Array(w384, w319, w318, w317, w316, w315, w314, w313, w312, w311, w310, w309, w308, w307) -> (w42:refnum<vi>[])
  n335 = control-ref of="BL Exp LB"() -> (w297:refnum<vi>)
  n336 = control-ref of="BL Exp LB 2"() -> (w296:refnum<vi>)
  n337 = control-ref of="BL Exp LB 3"() -> (w295:refnum<vi>)
  n338 = control-ref of="BL Exp LB 4"() -> (w278:refnum<vi>)
  n339 = control-ref of="BL Exp LB 5"() -> (w277:refnum<vi>)
  n340 = control-ref of="BL Exp LB 6"() -> (w198:refnum<vi>)
  n341 = control-ref of="BL Exp LB 7"() -> (w197:refnum<vi>)
  n342 = control-ref of="BL Exp LB 8"() -> (w196:refnum<vi>)
  n343 = Build Array (concatenate)(w116, w115, w114, w113, w15) -> (w75:refnum<vi>[])
  n344 = for {
    tunnel: w130 -> [w430] mode=indexing
    n345 = property class="Pict (strict)"(reference=w430, "Caption.Visible"=FALSE) -> ()  [unwired: 1 in, 2 out]
  }
  n346 = call "PH_Interaction.get Vision IDs on same Node.vi"("Cam Instances"=w107, "i ref in"="object ref") -> ("Vision System IDs"=w104:string[], "Vision Sytem IDs found"=w61:bool, "Cams instanciated on own system"=w103:bool)  [unwired: 1 in]
  n347 = Build Array(w297, w296, w295, w278, w277, w198, w197, w196) -> (w40:refnum<vi>[])
  n348 = Index Array(array=w104) -> (element=w106:string)  [unwired: 1 in]
  n349 = control-ref of="Force Sensor Instances"() -> (w14:refnum<vi>)
  n350 = control-ref of="Switch Instances"() -> (w11:refnum<vi>)
  n351 = control-ref of="Black Box Instances"() -> (w10:refnum<vi>)
  n352 = control-ref of="6P Switch Instances"() -> (w9:refnum<vi>)
  n353 = control-ref of="Switch GUI Instances"() -> (w8:refnum<vi>)
  n354 = control-ref of="Switch and 6P Instances"() -> (w7:refnum<vi>)
  n355 = control-ref of="Delete"() -> (w2:refnum<vi>)
  n356 = control-ref of="Ready for Shot"() -> (w72:refnum<vi>)
  n357 = Or(x=w103, y=w61) -> (x .or. y?=w3:bool)
  n358 = Select(t=w106, s=w61, f="N/A") -> (s? t:f=w70:string)
  n359 = Bundle By Name(cluster=T17 {"Vac GUI Refs"=[], "O2 GUI Refs"=[], "Ready for Shot"=refnum, "Boolean Condition Service Subscriber GUI Refs"=[], "Vision ID on same Node"="", "Picture Condition Service Subscriber GUI Refs"=[], "6P 4Q GUI Refs"=[], "Ref Switch GUI Instances"=refnum, "Ref 6P Switch Instances"=refnum, "Ref BB Instances"=refnum, "Ref Switch Instances"=refnum, "Ref Switch and 6P State Instances"=refnum, "Boolean Status Service Subscriber GUI Refs"=[], "Picture Status Service Subscriber GUI Refs"=[], "Force Sensor Instances"=refnum, "GUI Ref Delete"=refnum} ("PH_BL_Master GUI Refs"), "Force Sensor Instances"=w14, "Ref Switch Instances"=w11, "Ref BB Instances"=w10, "Ref 6P Switch Instances"=w9, "Ref Switch GUI Instances"=w8, "Ref Switch and 6P State Instances"=w7, "Vac GUI Refs"=w74, "O2 GUI Refs"=w73, "GUI Ref Delete"=w2, "Ready for Shot"=w72, "Boolean Condition Service Subscriber GUI Refs"=w71, "Picture Condition Service Subscriber GUI Refs"=w13, "6P 4Q GUI Refs"=w12, "Boolean Status Service Subscriber GUI Refs"=w75, "Picture Status Service Subscriber GUI Refs"=w6, "Vision ID on same Node"=w70) -> (w5:T17)
  n360 = control-ref of="Calibrator"() -> (w65:refnum<vi>)
  n361 = control-ref of="Igni MA 1: Heating off"() -> (w267:refnum<vi>)
  n362 = control-ref of="Igni MA 2: Heating off"() -> (w266:refnum<vi>)
  n363 = control-ref of="Igni MA 3: Heating off"() -> (w265:refnum<vi>)
  n364 = control-ref of="Igni MA 4: Heating off"() -> (w264:refnum<vi>)
  n365 = control-ref of="Igni MA 5: Heating off"() -> (w263:refnum<vi>)
  n366 = control-ref of="Igni FR: Heating off"() -> (w262:refnum<vi>)
  n367 = control-ref of="CoG"() -> (w66:refnum<vi>)
  n368 = control-ref of="PreAmp ok"() -> (w24:refnum<vi>)
  n369 = control-ref of="MainAmp ok"() -> (w25:refnum<vi>)
  n370 = control-ref of="fs Frontend ok"() -> (w26:refnum<vi>)
  n371 = control-ref of="ns Frontend ok"() -> (w27:refnum<vi>)
  n372 = control-ref of="PA ED ok"() -> (w28:refnum<vi>)
  n373 = control-ref of="In.-Box ok"() -> (w29:refnum<vi>)
  n374 = control-ref of="MAS ok"() -> (w30:refnum<vi>)
  n375 = control-ref of="Booster ok"() -> (w31:refnum<vi>)
  n376 = control-ref of="Mirrortower ok"() -> (w32:refnum<vi>)
  n377 = control-ref of="Compressor ok"() -> (w33:refnum<vi>)
  n378 = control-ref of="Experiment LB ok"() -> (w34:refnum<vi>)
  n379 = control-ref of="Laserlab ok"() -> (w35:refnum<vi>)
  n380 = control-ref of="Exp.-Shutters closed"() -> (w36:refnum<vi>)
  n381 = control-ref of="uOPA ok"() -> (w37:refnum<vi>)
  n382 = control-ref of="PHELIX_Beckhoff_Watchdog"() -> (w55:refnum<vi>)
  n383 = control-ref of="Intensity LB below Limit"() -> (w53:refnum<vi>)
  n384 = control-ref of="Intensity LL below Limit"() -> (w52:refnum<vi>)
  n385 = control-ref of="Vacuum no shotcond Comp LB"() -> (w51:refnum<vi>)
  n386 = control-ref of="PHELIX_Timing_Mode"() -> (w80:refnum<vi>)
  n387 = Build Array(w66, w65) -> (w23:refnum<vi>[])
  n388 = control-ref of="Exp: Shotmode"() -> (w59:refnum<vi>)
  n389 = control-ref of="LL: Shotmode"() -> (w58:refnum<vi>)
  n390 = control-ref of="Laserbay evacuated?"() -> (w57:refnum<vi>)
  n391 = control-ref of="Laserlab evacuated?"() -> (w56:refnum<vi>)
  n392 = control-ref of="HV room locked?"() -> (w54:refnum<vi>)
  n393 = Build Array(w267, w266, w265, w264, w263, w262) -> (w60:refnum<vi>[])
  n394 = control-ref of="Tab Control"() -> (w283:refnum<vi>)
  n395 = control-ref of="Laser enabled"() -> (w208:refnum<vi>)
  n396 = control-ref of="PreAmp enabled"() -> (w207:refnum<vi>)
  n397 = control-ref of="MainAmp enabled"() -> (w206:refnum<vi>)
  n398 = control-ref of="Emergency Off"() -> (w201:refnum<vi>)
  n399 = control-ref of="Shutter Exp 1"() -> (w202:refnum<vi>)
  n400 = control-ref of="Shutter Exp 2"() -> (w203:refnum<vi>)
  n401 = control-ref of="Shutter Exp 3"() -> (w204:refnum<vi>)
  n402 = control-ref of="Shutter Exp 4 (Z6)"() -> (w205:refnum<vi>)
  n403 = call "PH_Beamline.set start page.vi"("i ref in"="object ref", "Tab Control Ref"=w283, "error in (no error)"=w64) -> ("i ref out"=w69:refnum<vi>, "error out"=w68:errorcluster)  [unwired: 15 in]
  n404 = Bundle By Name(cluster=T16 {"Vision on this Node?"=FALSE, "Vision Knobs"=[], "GUI Refs"={"PA ok"=refnum, "MA ok"=refnum, "fs FE ok"=refnum, "ns FE ok"=refnum, "PA ED ok"=refnum, "MAS ok"=refnum, "Booster ok"=refnum, "Mirrortower ok"=refnum, "In.-Box ok"=refnum, "Compressor ok"=refnum, "Experiment LB ok"=refnum, "Experiment LL ok"=refnum, "PHELIX_Beckhoff_Watchdog"=refnum, "Shutters closed"=refnum, "uOPA ok"=refnum, "Vacuum no shotcond Comp LB"=refnum}, "PP Igni Heating GUI Refs"=[], "Refs BL PA"={"undelayed Line before Shutter"=[], "undelayed Line after Shutter"=[], "before Bypass"=[], "delayed Line before Shutter"=[], "delayed Line after Shutter"=[], "before Shutter Input"=[], "after Shutter Input"=[], "Bypass"=[], "before Shutter Exit"=[], "after Shutter Exit"=[], "to MA"=[], "to Lab"=[]}, "Refs BL MA"=[], "Refs BL MA-IB"=[], "Refs BL fs"=[], "Refs BL PA ED"=[], "Refs BL MAS"=[], "Refs BL Boo"=[], "Refs BL ns"=[], "Refs BL Mirrortower"=[], "Refs BL Compressor"=[], "Refs BL Exp LB"=[], "Refs BL LL"=[], "Refs BL uOPA"=[], "Ref Op Mode Exp LB"=refnum, "Ref Laserbay evacuated"=refnum, "Ref Op Mode Exp LL"=refnum, "Ref Laserlab evacuated"=refnum, "Ref HV room locked"=refnum, "Ref Bridge LB"=refnum, "Ref Bridge LL"=refnum} ("PH Beamline GUI Refs"), "GUI Refs.PA ok"=w24, "GUI Refs.MA ok"=w25, "GUI Refs.fs FE ok"=w26, "GUI Refs.ns FE ok"=w27, "GUI Refs.PA ED ok"=w28, "GUI Refs.In.-Box ok"=w29, "GUI Refs.MAS ok"=w30, "GUI Refs.Booster ok"=w31, "GUI Refs.Mirrortower ok"=w32, "GUI Refs.Compressor ok"=w33, "GUI Refs.Experiment LB ok"=w34, "GUI Refs.Experiment LL ok"=w35, "GUI Refs.Shutters closed"=w36, "GUI Refs.uOPA ok"=w37, "Refs BL PA"=w38, "Refs BL MA"=w39, "Refs BL Exp LB"=w40, "Refs BL Compressor"=w41, "Refs BL MA-IB"=w42, "Refs BL fs"=w43, "Refs BL PA ED"=w44, "Refs BL MAS"=w45, "Refs BL Boo"=w46, "Refs BL ns"=w47, "Refs BL Mirrortower"=w48, "Refs BL LL"=w49, "Refs BL uOPA"=w50, "Ref Op Mode Exp LB"=w59, "Ref Op Mode Exp LL"=w58, "Ref Laserbay evacuated"=w57, "Ref Laserlab evacuated"=w56, "GUI Refs.PHELIX_Beckhoff_Watchdog"=w55, "Ref HV room locked"=w54, "Ref Bridge LB"=w53, "Ref Bridge LL"=w52, "GUI Refs.Vacuum no shotcond Comp LB"=w51, "PP Igni Heating GUI Refs"=w60, "Vision Knobs"=w23, "Vision on this Node?"=w3) -> (w22:T16)
  n405 = Bundle By Name(cluster=T18 {"Laser"=refnum, "PreAmp"=refnum, "MainAmp"=refnum, "Emergency Off"=refnum, "Exp 1"=refnum, "Exp 2"=refnum, "Exp 3"=refnum, "Exp 4"=refnum, "Timing Mode GUI Ref"=refnum} ("Color GUI Refs"), "Laser"=w208, "PreAmp"=w207, "MainAmp"=w206, "Emergency Off"=w201, "Exp 1"=w202, "Exp 2"=w203, "Exp 3"=w204, "Exp 4"=w205, "Timing Mode GUI Ref"=w80) -> (w1:T18)
  n406 = call "PH_Class.Register Event.vi"("i ref in"=w69, "error in (no error)"=w68) -> ("i ref out"=w78:refnum<vi>, "Event Registration Refnum"=w67:refnum<event-registration>, "error out"=w77:errorcluster)  [unwired: 15 in]
  n407 = while {
    tunnel: w78 -> [w438]
    tunnel: [w437] -> w327
    tunnel: w77 -> [w440]
    tunnel: [w439] -> w326
    tunnel: [w435] -> w79
    tunnel: w67 -> [w434]
    tunnel: w22 -> [w433]
    tunnel: w1 -> [w432]
    tunnel: w5 -> [w431]
    stop <- w436 stop-if-true
    n408 = event shown="[6] \"PA_Input_2_Beam_6PWpGUI\", \"MA_MM3_6PGUI\", \"MA_Inject_C_NF2GUI\", \"PA_MM_C_Input_NF2GUI\", \"PA_MM_P_Input_NF2GUI\", \"MA_Inject_P_6PGUI\", \"MA_MM9_6PGUI\", \"MA_MM8_6PGUI\", \"PA_C_MA_6PGUI\", \"Compressor_Grating_2_Tip+Tilt_6PGUI\", \"Compressor_Grating_2_6PGUI\", \"Compressor_Grating_1_Tip+Tilt_6PGUI\", \"Compressor_Grating_1_6PGUI\", \"Compressor_LM_6PGUI\", \"Compressor_Turnbox_2_Trans_6PGUI\", \"Compressor_Turnbox_2_6PGUI\", \"Compressor_Turnbox_1_Trans_6PGUI\", \"Compressor_Turnbox_1_6PGUI\", \"Experiment_Targetmanipulator_TURN_6PGUI\", \"Experiment_Targetmanipulator_TRANS_6PGUI\", \"Experiment_Targetmanipulator_6PGUI\", \"fs_Stretcher_6PGUI\", \"fs_RR_Cavity_NF2GUI\", \"PA_Input_Delay_6PGUI\", \"PA_LL_C_6PGUI\", \"PA_LL_P_6PGUI\", \"LL_Comp_C_6PGUI\", \"LL_Comp_P_6PGUI\", \"LL_Comp_Grating_Rot_6PGUI\", \"LL_Comp_Length_6PGUI\", \"MAS_Beam_Fine_Attenuator_6PWpGUI\", \"MAS_Discrete_Spectro_Rev6PGUI\", \"fs_WP_Exit_6PWpGUI\", \"ns_WP_RR_6PWpGUI\", \"COS_WP_6PWpGUI\", \"PA_ML_T3_Exit_6P4QGUI\", \"PA_PiH_VSF2_6PGUI\", \"PA_PiH_VSF4_6PGUI\", \"PA_WP_Exit_6PWpGUI\", \"YLF_WP_6PWpGUI\", \"PA_SA_6P4QGUI\", \"MA_ML_In_6P4QGUI\", \"MA_MM2_6PGUI\", \"MA_MM4_6PGUI\", \"uOPA_Pump_WP_6PWpGUI\", \"MA_MM1_6P4QGUI\", \"MA_MM1_Bend_6P4QGUI\": Mouse Up" {
      selector: w434 -> [_ _ _ _ _ _ _ _ _ _ _ _ _ _ _ _ _ _ _ _ _ _]
      dyn-events: [_ _ _ _ _ _ _ _ _ _ _ _ _ _ _ _ _ _ _ _ _ _] -> w435
      timeout: _ -> [_ _ _ _ _ _ _ _ _ _ _ _ _ _ _ _ _ _ _ _ _ _]
      tunnel: w438 -> [w447 w452 w453 w475 w537 w614 w625 w649 w657 w668 w677 w685 w693 w698 w706 w716 w728 _ w792 w834 w851 w863]
      tunnel: w440 -> [w442 w451 w455 w477 w538 w622 w624 w651 w659 w667 w676 w683 w691 w701 w709 w719 w725 _ w798 w837 w854 w862]
      tunnel: [w446 w450 w454 w472 w529 w617 w628 w653 w661 w670 w678 w686 w694 w702 w710 w715 w731 _ w797 w836 w852 w865] -> w439
      tunnel: [w445 w449 w453 w471 w531 w618 w629 w654 w662 w671 w679 w687 w695 w703 w711 w714 w730 _ w791 w835 w851 w864] -> w437
      tunnel: ["Delete" _ _ _ _ _ _ _ _ _ _ _ _ _ _ _ _ _ _ _ _ _] -> w436
      tunnel: w433 -> [_ _ _ _ _ _ _ _ _ _ _ _ _ _ _ _ _ _ _ _ _ w858]
      tunnel: w432 -> [_ _ _ _ _ _ _ _ _ _ _ _ _ _ _ _ _ _ _ _ _ w856]
      tunnel: w431 -> [_ _ _ _ _ _ _ _ _ _ _ _ _ _ _ _ _ _ _ _ _ w857]
      event "Delete": Value Change {
        n409 = event-data() -> ()  [unwired: 1 in, 1 out]
        n410 = call "PH_GUI.Manager Close.vi"("i ref in"=w447, "error in"=w442) -> ("i ref out"=w443:refnum<vi>, "error out"=w441:errorcluster)  [unwired: 16 in]
        n411 = call "CSObj.open front panel.vi"("i ref in"=w443, "frontPanelOpen"=FALSE ("front panel open"), "error in (no error)"=w441) -> ("i ref out"=w445:refnum<vi>, "error out"=w446:errorcluster)  [unwired: 15 in]
      }
      event "Minimize": Value Change {
        n412 = event-data() -> ()  [unwired: 1 in, 1 out]
        n413 = call "PH_GUI.Manager Minimize.vi"("i ref in"=w452, "error in"=w451) -> ("i ref out"=w449:refnum<vi>, "error out"=w450:errorcluster)  [unwired: 16 in]
      }
      event "Remote Desktop Connection": Value Change {
        n414 = event-data() -> ()  [unwired: 1 in, 1 out]
        n415 = call "PH_Connection.select PCS Node.vi"("error in"=w455) -> ("string out"=w456:string, "error out"=w457:errorcluster)  [unwired: 17 in]
        n416 = case shown="Default" w456 {
          selector: w456 -> [_ w459]
          tunnel: w457 -> [w458 w461]
          tunnel: [w458 w460] -> w454
          frame "", "N/A" {
          }
          frame Default {
            n417 = Concatenate Strings("mstsc " ("command line"), w459) -> (w463:string)
            n418 = call <vilib>:"System Exec.vi"("wait until completion? (T)"=FALSE, "error in (no error)"=w461, "command line"=w463) -> ("error out"=w460:errorcluster)  [unwired: 5 in, 3 out]
          }
        }
      }
      event Mouse Up {
        n419 = event-data() -> ("CtlRef"=w476:refnum<vi>)  [unwired: 1 in]
        n420 = property class="Pict (strict)"(reference=w476, error in=w477) -> (error out=w474:errorcluster, "Label.Text"=w465:string)  [unwired: 1 out]
        n421 = call "PH_BL-Master.get Picture Status Service Subscriber Status by Name.vi"("i ref in"=w475, "Picture Status Subscriber Instance"=w465, "error in (no error)"=w474) -> ("i ref out"=w466:refnum<vi>, "on/true/in?"=w473:bool, "error out"=w469:errorcluster)  [unwired: 7 in, 7 out]
        n422 = Not(x=w473) -> (.not. x?=w470:bool)
        n423 = case shown="False" w470 {
          tunnel: [w482 w486] -> w467
          tunnel: [w481 w487] -> w468
          tunnel: w465 -> [w480 w485]
          tunnel: w469 -> [w479 w483]
          tunnel: w466 -> [w478 w484]
          frame False {
            n424 = call "PH_Switch.evt false.vi"("i ref in"=w478, "Instance"=w480, "error in (no error)"=w479) -> ("i ref out"=w482:refnum<vi>, "error out"=w481:errorcluster)  [unwired: 15 in]
          }
          frame True {
            n425 = call "PH_Switch.evt true.vi"("i ref in"=w484, "Instance"=w485, "error in (no error)"=w483) -> ("i ref out"=w486:refnum<vi>, "error out"=w487:errorcluster)  [unwired: 15 in]
          }
        }
        n426 = case shown="\"MA_InB_IM_In_Switch\"" w465 {
          tunnel: w468 -> [w489 w491 w508]
          tunnel: [w489 w495 w509] -> w472
          tunnel: w467 -> [w488 w492 w511]
          tunnel: [w488 w494 w510] -> w471
          tunnel: w470 -> [_ w490 w506]
          frame Default {
          }
          frame "MA_InB_IM_Out_Switch" {
            n427 = case shown="False" w490 {
              tunnel: w492 -> [w500 w505]
              tunnel: [w499 w502] -> w494
              tunnel: w491 -> [w498 w504]
              tunnel: [w497 w503] -> w495
              tunnel: T9 "MA_InB_DP_Out_Switch" ("Switch") -> [w496 w501]
              frame False {
                n428 = call "PH_Switch.evt false.vi"("i ref in"=w500, "Instance"=w496, "error in (no error)"=w498) -> ("i ref out"=w499:refnum<vi>, "error out"=w497:errorcluster)  [unwired: 15 in]
              }
              frame True {
                n429 = call "PH_Switch.evt true.vi"("i ref in"=w505, "Instance"=w501, "error in (no error)"=w504) -> ("i ref out"=w502:refnum<vi>, "error out"=w503:errorcluster)  [unwired: 15 in]
              }
            }
          }
          frame "MA_InB_IM_In_Switch" {
            n430 = case shown="False" w506 {
              tunnel: w511 -> [w516 w521]
              tunnel: [w515 w518] -> w510
              tunnel: w508 -> [w514 w520]
              tunnel: [w513 w519] -> w509
              tunnel: T9 "MA_InB_DP_In_Switch" ("Switch") -> [w512 w517]
              frame False {
                n431 = call "PH_Switch.evt false.vi"("i ref in"=w516, "Instance"=w512, "error in (no error)"=w514) -> ("i ref out"=w515:refnum<vi>, "error out"=w513:errorcluster)  [unwired: 15 in]
              }
              frame True {
                n432 = call "PH_Switch.evt true.vi"("i ref in"=w521, "Instance"=w517, "error in (no error)"=w520) -> ("i ref out"=w518:refnum<vi>, "error out"=w519:errorcluster)  [unwired: 15 in]
              }
            }
          }
        }
      }
      event "BL-Z6-Beamdump", "MainAmp_Flowbox_off", "FR+MT_Flowbox_off", "MA_InB_DP_In_Switch", "MA_InB_DP_Out_Switch", "Shutter_Exp_Laserbay", "Shutter_Laserlab": Value Change {
        n433 = event-data() -> ("CtlRef"=w533:refnum<vi>, "OldVal"=w526:bool)  [unwired: 1 in]
        n434 = property class="Bool (strict)"(reference=w533, error in=w538, "Value"=w526) -> (error out=w536:errorcluster, "Label.Text"=w524:string)  [unwired: 1 out]
        n435 = call "PH_BL-Master.get Boolean Status Service Subscriber Status by Name.vi"("i ref in"=w537, "Status Subscriber Instance"=w524, "error in (no error)"=w536) -> ("i ref out"=w523:refnum<vi>, "on/true/in?"=w535:bool, "error out"=w522:errorcluster)  [unwired: 7 in, 7 out]
        n436 = Not(x=w535) -> (.not. x?=w534:bool)
        n437 = case shown="\"Shutter_Laserlab\"" w524 {
          selector: w524 -> [w559 w569 w573 w585 w603]
          tunnel: w522 -> [w561 w566 w577 w581 w599]
          tunnel: [w561 w565 w576 w582 w597] -> w530
          tunnel: w523 -> [w560 w568 w575 w584 w602]
          tunnel: [w560 w567 w574 w583 w601] -> w532
          tunnel: [w559 w569 w573 w585 w603] -> w528
          tunnel: w534 -> [w558 w563 w571 w580 w598]
          tunnel: [w558 w563 w571 w580 w598] -> w527
          tunnel: [TRUE ("on/true/in?") w564 w572 TRUE ("on/true/in?") TRUE ("on/true/in?")] -> w525
          frame Default {
          }
          frame "Shutter_Laserlab" {
            n438 = call "PH_BL-Master.get Boolean Status Service Subscriber Status by Name.vi"("i ref in"=w568, "Status Subscriber Instance"=T6 "Shutter_Laserlab_Interlock" ("Switch GUI"), "error in (no error)"=w566) -> ("i ref out"=w567:refnum<vi>, "on/true/in?"=w564:bool, "error out"=w565:errorcluster)  [unwired: 7 in, 7 out]
          }
          frame "Shutter_Exp_Laserbay" {
            n439 = call "PH_BL-Master.get Boolean Status Service Subscriber Status by Name.vi"("i ref in"=w575, "Status Subscriber Instance"=T6 "Shutter_Exp_Laserbay_Interlock" ("Switch GUI"), "error in (no error)"=w577) -> ("i ref out"=w574:refnum<vi>, "on/true/in?"=w572:bool, "error out"=w576:errorcluster)  [unwired: 7 in, 7 out]
          }
          frame "MA_InB_DP_In_Switch" {
            n440 = case shown="False" w580 {
              tunnel: [w590 w594] -> w583
              tunnel: [w589 w595] -> w582
              tunnel: T9 "MA_InB_IM_In_Switch" ("Switch") -> [w588 w593]
              tunnel: w581 -> [w587 w591]
              tunnel: w584 -> [w586 w592]
              frame False {
                n441 = call "PH_Switch.evt false.vi"("i ref in"=w586, "Instance"=w588, "error in (no error)"=w587) -> ("i ref out"=w590:refnum<vi>, "error out"=w589:errorcluster)  [unwired: 15 in]
              }
              frame True {
                n442 = call "PH_Switch.evt true.vi"("i ref in"=w592, "Instance"=w593, "error in (no error)"=w591) -> ("i ref out"=w594:refnum<vi>, "error out"=w595:errorcluster)  [unwired: 15 in]
              }
            }
          }
          frame "MA_InB_DP_Out_Switch" {
            n443 = case shown="False" w598 {
              tunnel: [w608 w612] -> w601
              tunnel: [w607 w613] -> w597
              tunnel: T9 "MA_InB_IM_Out_Switch" ("Switch") -> [w606 w611]
              tunnel: w599 -> [w605 w609]
              tunnel: w602 -> [w604 w610]
              frame False {
                n444 = call "PH_Switch.evt false.vi"("i ref in"=w604, "Instance"=w606, "error in (no error)"=w605) -> ("i ref out"=w608:refnum<vi>, "error out"=w607:errorcluster)  [unwired: 15 in]
              }
              frame True {
                n445 = call "PH_Switch.evt true.vi"("i ref in"=w610, "Instance"=w611, "error in (no error)"=w609) -> ("i ref out"=w612:refnum<vi>, "error out"=w613:errorcluster)  [unwired: 15 in]
              }
            }
          }
        }
        n446 = case shown="True" w525 {
          tunnel: w532 -> [w540 w546]
          tunnel: [w540 w545] -> w531
          tunnel: w530 -> [w539 w544]
          tunnel: [w539 w543] -> w529
          tunnel: w528 -> [_ w542]
          tunnel: w527 -> [_ w541]
          frame False {
          }
          frame True {
            n447 = case shown="False" w541 {
              tunnel: [w551 w555] -> w545
              tunnel: [w550 w556] -> w543
              tunnel: w542 -> [w549 w554]
              tunnel: w544 -> [w548 w552]
              tunnel: w546 -> [w547 w553]
              frame False {
                n448 = call "PH_Switch.evt false.vi"("i ref in"=w547, "Instance"=w549, "error in (no error)"=w548) -> ("i ref out"=w551:refnum<vi>, "error out"=w550:errorcluster)  [unwired: 15 in]
              }
              frame True {
                n449 = call "PH_Switch.evt true.vi"("i ref in"=w553, "Instance"=w554, "error in (no error)"=w552) -> ("i ref out"=w555:refnum<vi>, "error out"=w556:errorcluster)  [unwired: 15 in]
              }
            }
          }
        }
      }
      event "COS_Sensitivity_Switch", "Calorimeter_Switch": Value Change {
        n450 = event-data() -> ("CtlRef"=w621:refnum<vi>, "OldVal"=w620:bool)  [unwired: 1 in]
        n451 = property class="Bool (strict)"(reference=w621, error in=w622, "Value"=w620) -> (error out=w615:errorcluster, "Label.Text"=w616:string)  [unwired: 1 out]
        n452 = call "PH_Sixpack_Switch.evt move.vi"("i ref in"=w614, "Instance"=w616, "Move"=TRUE, "error in (no error)"=w615) -> ("i ref out"=w618:refnum<vi>, "error out"=w617:errorcluster)  [unwired: 14 in]
      }
      event Mouse Up {
        n453 = event-data() -> ("CtlRef"=w627:refnum<vi>)  [unwired: 1 in]
        n454 = property class="Pict (strict)"(reference=w627, error in=w624) -> (error out=w623:errorcluster, "Label.Text"=w626:string)  [unwired: 1 out]
        n455 = case shown="Default" w626 {
          selector: w626 -> [w631 w642]
          tunnel: [w635 w646] -> w629
          tunnel: [w633 w645] -> w628
          tunnel: w625 -> [w636 w644]
          tunnel: w623 -> [w634 w643]
          frame "MA_PiH_Vert_NFGUI" {
            n456 = Build Array(w631, T20 "MA_PiH_Hor_NFGUI" ("Motion GUI Instances")) -> (w632:T20[])
            n457 = for {
              shift-right: [w640] -> w635
              shift-left: w636 -> [w641]
              shift-right: [w638] -> w633
              shift-left: w634 -> [w639]
              tunnel: w632 -> [w637] mode=indexing
              n458 = call "PH_Interaction.Open or Create Singleton Instance.vi"("i ref in"=w641, "Instance to create or to open"=w637, "error IO"=w639) -> ("i ref out"=w640:refnum<vi>, "error out"=w638:errorcluster)  [unwired: 15 in]
            }
          }
          frame Default {
            n459 = call "PH_Interaction.Open or Create Singleton Instance.vi"("i ref in"=w644, "Instance to create or to open"=w642, "error IO"=w643) -> ("i ref out"=w646:refnum<vi>, "error out"=w645:errorcluster)  [unwired: 15 in]
          }
        }
      }
      event "Shutter_Exp_Laserbay_Interlock", "Shutter_Laserlab_Interlock": Value Change {
        n460 = event-data() -> ("CtlRef"=w652:refnum<vi>, "OldVal"=w647:bool)  [unwired: 1 in]
        n461 = property class="Bool (strict)"(reference=w652, error in=w651, "Value"=w647) -> (error out=w648:errorcluster, "Label.Text"=w650:string)  [unwired: 1 out]
        n462 = call "PH_Interaction.Open or Create Singleton Instance.vi"("i ref in"=w649, "Instance to create or to open"=w650, "error IO"=w648) -> ("i ref out"=w654:refnum<vi>, "error out"=w653:errorcluster)  [unwired: 15 in]
      }
      event "MM1_ForceSensor": Value Change {
        n463 = event-data() -> ("CtlRef"=w660:refnum<vi>, "OldVal"=w655:bool)  [unwired: 1 in]
        n464 = property class="Bool (strict)"(reference=w660, error in=w659, "Value"=w655) -> (error out=w656:errorcluster, "Label.Text"=w658:string)  [unwired: 1 out]
        n465 = call "PH_Interaction.Open or Create Singleton Instance.vi"("i ref in"=w657, "Instance to create or to open"=w658, "error IO"=w656) -> ("i ref out"=w662:refnum<vi>, "error out"=w661:errorcluster)  [unwired: 15 in]
      }
      event Mouse Up {
        n466 = event-data() -> ("CtlRef"=w669:refnum<vi>)  [unwired: 1 in]
        n467 = property class="Pict (strict)"(reference=w669, error in=w667) -> (error out=w666:errorcluster, "Label.Text"=w664:string)  [unwired: 1 out]
        n468 = Match Pattern(string=w664, regular expression="::") -> (after substring=w663:string)  [unwired: 1 in, 3 out]
        n469 = call "PH_Interaction.Open or Create Singleton Instance.vi"("i ref in"=w668, "Instance to create or to open"=w663, "error IO"=w666) -> ("i ref out"=w671:refnum<vi>, "error out"=w670:errorcluster)  [unwired: 15 in]
      }
      event "PA_Exit_Powermeter", "MAS_Powermeter", "ns_Exit_Powermeter", "uOPA_Pump_Powermeter": Value Change {
        n470 = event-data() -> ("CtlRef"=w674:refnum<vi>, "OldVal"=w672:bool)  [unwired: 1 in]
        n471 = property class="Bool (strict)"(reference=w674, error in=w676, "Value"=w672) -> (error out=w675:errorcluster, "Label.Text"=w673:string)  [unwired: 1 out]
        n472 = call "PH_Interaction.Open or Create Singleton Instance.vi"("i ref in"=w677, "Instance to create or to open"=w673, "error IO"=w675) -> ("i ref out"=w679:refnum<vi>, "error out"=w678:errorcluster)  [unwired: 15 in]
      }
      event "ns_Nearfield_Ring_Exit_Cam", "ns_Farfield_Ring_Exit_Cam", "fs_Nearfield_Frontend_Cam", "PA_Nearfield_Input_Cam", "PA_Farfield_Input_Cam", "PA_Nearfield_Exit_Cam", "PA_Farfield_Exit_Cam", "MA_Nearfield_PiH_in_Cam", "MA_Nearfield_PiH_out_Cam", "MAS_Nearfield_Cam", "MAS_Farfield_High_Res_Cam", "MA_Alignment_Cam", "MA_Inject_In_Cam", "PA_MA_Bridge_Input_Cam", "COS_FF_Cam", "COS_NF_Cam", "PA_LL_Input_Cam", "COS_SSAC_Cam", "PA_LL_Output_Cam", "LL_Comp_FF_Cam", "LL_Comp_Input_Cam", "LL_SSAC_Cam", "MAS_SHS_Cam", "MAS_FF_HamamatsuCam", "uOPA_Regen_Cam", "PA_SHS_Input_Cam", "PA_SHS_Exit_Cam": Value Change {
        n473 = event-data() -> ("CtlRef"=w682:refnum<vi>, "OldVal"=w680:bool)  [unwired: 1 in]
        n474 = property class="Bool (strict)"(reference=w682, error in=w683, "Value"=w680) -> (error out=w684:errorcluster, "Label.Text"=w681:string)  [unwired: 1 out]
        n475 = call "PH_Interaction.Open or Create Singleton Instance.vi"("i ref in"=w685, "Instance to create or to open"=w681, "error IO"=w684) -> ("i ref out"=w687:refnum<vi>, "error out"=w686:errorcluster)  [unwired: 15 in]
      }
      event "MAS_OO_Spectrometer", "fs_OO_Spectrometer", "uOPA_Pump_OO_Spectrometer": Value Change {
        n476 = event-data() -> ("CtlRef"=w690:refnum<vi>, "OldVal"=w688:bool)  [unwired: 1 in]
        n477 = property class="Bool (strict)"(reference=w690, error in=w691, "Value"=w688) -> (error out=w692:errorcluster, "Label.Text"=w689:string)  [unwired: 1 out]
        n478 = call "PH_Interaction.Open or Create Singleton Instance.vi"("i ref in"=w693, "Instance to create or to open"=w689, "error IO"=w692) -> ("i ref out"=w695:refnum<vi>, "error out"=w694:errorcluster)  [unwired: 15 in]
      }
      event "ns_Nearfield_Ring_Exit_ImageOperator", "ns_Farfield_Ring_Exit_ImageOperator", "fs_Nearfield_Frontend_ImageOperator", "PA_Nearfield_Input_ImageOperator", "PA_Farfield_Input_ImageOperator", "PA_Nearfield_Exit_ImageOperator", "PA_Farfield_Exit_ImageOperator", "MA_Alignment_ImageOperator", "MA_Nearfield_PiH_in_ImageOperator", "MA_Nearfield_PiH_out_ImageOperator", "MAS_Nearfield_ImageOperator", "MAS_Farfield_High_Res_ImageOperator", "MA_Inject_In_ImageOperator": Value Change {
        n479 = event-data() -> ("CtlRef"=w699:refnum<vi>, "OldVal"=w696:bool)  [unwired: 1 in]
        n480 = property class="Bool (strict)"(reference=w699, error in=w701, "Value"=w696) -> (error out=w700:errorcluster, "Label.Text"=w697:string)  [unwired: 1 out]
        n481 = call "PH_Interaction.Open or Create Singleton Instance.vi"("i ref in"=w698, "Instance to create or to open"=w697, "error IO"=w700) -> ("i ref out"=w703:refnum<vi>, "error out"=w702:errorcluster)  [unwired: 15 in]
      }
      event "COS-SSAC", "LL-SSAC": Value Change {
        n482 = event-data() -> ("CtlRef"=w707:refnum<vi>, "OldVal"=w704:bool)  [unwired: 1 in]
        n483 = property class="Bool (strict)"(reference=w707, error in=w709, "Value"=w704) -> (error out=w708:errorcluster, "Label.Text"=w705:string)  [unwired: 1 out]
        n484 = call "PH_Interaction.Open or Create Singleton Instance.vi"("i ref in"=w706, "Instance to create or to open"=w705, "error IO"=w708) -> ("i ref out"=w711:refnum<vi>, "error out"=w710:errorcluster)  [unwired: 15 in]
      }
      event "PA_PC_WP_BB", "PA_Exit_Shut_BB", "PA_ED_FILT1_BB", "MAS_Attenuator_1_BB", "MA_Shut_AlignCam_BB", "MA_Diffusor_Inject_In_BB", "NS_Shut_PA_BB", "FS_Shut_PA_BB", "PA_Shut_Input_BB", "COS_Filt1_BB", "PA_PC_WP_2_BB", "PA_LL_CH_Input_BB", "PA_delayed_BB", "PA_non_delayed_BB", "PA_LL_CH_Output_BB", "LL_Shut_Comp_Input_BB", "LL_Shut_Comp_FF_BB", "LL_Shut_Comp_Output_BB": Value Change {
        n485 = event-data() -> ("CtlRef"=w718:refnum<vi>, "OldVal"=w712:bool)  [unwired: 1 in]
        n486 = property class="Bool (strict)"(reference=w718, error in=w719, "Value"=w712) -> (error out=w717:errorcluster, "Label.Text"=w713:string)  [unwired: 1 out]
        n487 = call "PH_BlackBox.evt start move.vi"("i ref in"=w716, "Instance"=w713, "error in (no error)"=w717) -> ("i ref out"=w714:refnum<vi>, "error out"=w715:errorcluster)  [unwired: 15 in]
      }
      event Mouse Up {
        n488 = event-data() -> ("CtlRef"=w734:refnum<vi>)  [unwired: 1 in]
        n489 = call "PH_Beamline.get i attribute.vi"("i ref in"=w728, "error in (no error)"=w725) -> ("i ref out"=w727:refnum<vi>, "i attribute"=w726:T22, "error out"=w724:errorcluster)  [unwired: 15 in]
        n490 = Unbundle By Name(w726) -> ("Status Subscriber Information.PA PC WP 2"=w720:T24, "Status Subscriber Information.fs Swich YLF"=w721:T24, "Status Subscriber Information.PA PC WP"=w722:T24)
        n491 = property class="Pict (strict)"(reference=w734, error in=w724) -> (error out=w723:errorcluster, "Label.Text"=w729:string)  [unwired: 1 out]
        n492 = case shown="\"FS_Switch_YLF_BB\"" w729 {
          tunnel: [w736 w754] -> w733
          tunnel: [w735 w756] -> w732
          tunnel: w723 -> [w736 w764]
          tunnel: w727 -> [w735 w763]
          tunnel: w722 -> [_ w739]
          tunnel: w721 -> [_ w738]
          tunnel: w720 -> [_ w737]
          frame Default {
          }
          frame "FS_Switch_YLF_BB" {
            w742 = T27[] [2, 1] items=["no info", "off/false/out", "on/true/in", "Failure", "Alarm", "Status 1", "Status 2", "Status 3"] ("y")
            w743 = T27[] [1, 2] items=["no info", "off/false/out", "on/true/in", "Failure", "Alarm", "Status 1", "Status 2", "Status 3"] ("y")
            n493 = call "PH_BL-Master.get Status of Status Service Subscriber.vi"("i ref in"=w763, "Wanted Status Subscriber Information"=w739, "error in (no error)"=w764) -> ("i ref out"=w766:refnum<vi>, "Status"=w762:T27, "error out"=w765:errorcluster)  [unwired: 11 in, 3 out]
            n494 = call "PH_BL-Master.get Status of Status Service Subscriber.vi"("i ref in"=w766, "Wanted Status Subscriber Information"=w738, "error in (no error)"=w765) -> ("i ref out"=w747:refnum<vi>, "Status"=w744:T27, "error out"=w749:errorcluster)  [unwired: 11 in, 3 out]
            n495 = Build Array(w744, w762) -> (w761:T27[])
            n496 = call "PH_BL-Master.get Status of Status Service Subscriber.vi"("i ref in"=w747, "Wanted Status Subscriber Information"=w737, "error in (no error)"=w749) -> ("i ref out"=w746:refnum<vi>, "Status"=w745:T27, "error out"=w748:errorcluster)  [unwired: 11 in, 3 out]
            n497 = Equal?(x=w761, y=w743) -> (x = y?=w760:bool)
            n498 = Equal?(x=w761, y=w742) -> (x = y?=w759:bool)
            n499 = Build Array(w744, w745) -> (w753:T27[])
            n500 = Or(x=w760, y=w759) -> (x .or. y?=w758:bool)
            n501 = Equal?(x=w753, y=w743) -> (x = y?=w752:bool)
            n502 = Equal?(x=w753, y=w742) -> (x = y?=w751:bool)
            n503 = Or(x=w752, y=w751) -> (x .or. y?=w750:bool)
            n504 = case shown="True" w758 {
              tunnel: w748 -> [w774 w780]
              tunnel: [w774 w779] -> w755
              tunnel: w746 -> [w775 w778]
              tunnel: [w775 w777] -> w757
              tunnel: T7 "PA_PC_WP_BB" ("Black Box Instance") -> [_ w776]
              frame False {
              }
              frame True {
                n505 = call "PH_BlackBox.evt start move.vi"("i ref in"=w778, "Instance"=w776, "error in (no error)"=w780) -> ("i ref out"=w777:refnum<vi>, "error out"=w779:errorcluster)  [unwired: 15 in]
              }
            }
            n506 = case shown="True" w750 {
              tunnel: w755 -> [w767 w773]
              tunnel: [w767 w772] -> w754
              tunnel: w757 -> [w768 w771]
              tunnel: [w768 w770] -> w756
              tunnel: T7 "PA_PC_WP_2_BB" ("Black Box Instance") -> [_ w769]
              frame False {
              }
              frame True {
                n507 = call "PH_BlackBox.evt start move.vi"("i ref in"=w771, "Instance"=w769, "error in (no error)"=w773) -> ("i ref out"=w770:refnum<vi>, "error out"=w772:errorcluster)  [unwired: 15 in]
              }
            }
          }
        }
        n508 = call "PH_BlackBox.evt start move.vi"("i ref in"=w732, "Instance"=w729, "error in (no error)"=w733) -> ("i ref out"=w730:refnum<vi>, "error out"=w731:errorcluster)  [unwired: 15 in]
      }
      event "Hop 1", "Hop 2", "Hop 3", "Hop 4", "Hop 5", "Hop 6", "Hop 7", "Hop 8", "Hop 9", "Hop 10", "Hop 11", "Hop 12", "Hop 13", "Hop 14", "Hop 15", "Hop 16", "Hop 17", "Hop 18", "Hop 19", "Hop 20", "Hop 21", "Hop 22", "Hop 23", "Hop 24": Value Change {
        n509 = event-data() -> ("CtlRef"=w785:refnum<vi>)  [unwired: 1 in]
        n510 = property on="Tab Control" class="TabCtl (strict)"() -> ("Pages"=w784:refnum<vi>[])  [unwired: 2 in, 2 out]
        n511 = for {
          tunnel: [w788] -> w783 mode=indexing
          tunnel: w784 -> [w787] mode=indexing
          n512 = property class="Page"(reference=w787) -> ("Page Label"=w788:string)  [unwired: 1 in, 2 out]
        }
        n513 = property class="Bool"(reference=w785) -> ("Boolean Text.Text"=w782:string)  [unwired: 1 in, 2 out]
        n514 = Search 1D Array(1D array=w783, element=w782) -> (index of element=w781:i32)  [unwired: 1 in]
        n515 = case shown="Default" w781 {
          selector: w781 -> [_ w786]
          frame -1 {
          }
          frame Default {
            n516 = property on="Tab Control" class="TabCtl (strict)"("Value"=w786) -> ()  [unwired: 2 in, 2 out]
          }
        }
      }
      event "Image Statistician", "Calibrator", "PCS Main", "CoG", "Z6 Main", "Z6 Beamline": Value Change {
        n517 = event-data() -> ("CtlRef"=w796:refnum<vi>)  [unwired: 1 in]
        n518 = property class="Bool"(reference=w796, error in=w798) -> (error out=w790:errorcluster, "Label.Text"=w795:string)  [unwired: 1 out]
        n519 = case shown="\"CoG\"" w795 {
          tunnel: [T21."None" ("Instance to create or open") T21."PCS Main" ("Instance to create or open") T21."Z6 Main" ("Instance to create or open") T21."Z6 Beamline" ("Instance to create or open") T21."Image Statistician" ("Instance to create or open") T21."Image Center of Gravity" ("Instance to create or open") T21."Image Calibrator" ("Instance to create or open")] -> w794
          tunnel: ["N/A" ("Vision ID on same Node") "N/A" "N/A" "N/A" "N/A" w819 w826] -> w793
          tunnel: w790 -> [w800 w803 w807 w811 w815 w822 w831]
          tunnel: w792 -> [w801 w804 w808 w812 w816 w823 w830]
          tunnel: [w801 w804 w808 w812 w816 w821 w829] -> w791
          tunnel: [w800 w803 w807 w811 w815 w820 w828] -> w789
          frame Default {
          }
          frame "PCS Main" {
          }
          frame "Z6 Main" {
          }
          frame "Z6 Beamline" {
          }
          frame "Image Statistician" {
          }
          frame "CoG" {
            n520 = call "PH_BL-Master.get i attribute.vi"("i ref in"=w823, "error in (no error)"=w822) -> ("i ref out"=w821:refnum<vi>, "i attribute"=w824:T28, "error out"=w820:errorcluster)  [unwired: 15 in]
            n521 = Unbundle By Name(w824) -> ("Vision ID on same Node"=w819:string)
          }
          frame "Calibrator" {
            n522 = call "PH_BL-Master.get i attribute.vi"("i ref in"=w830, "error in (no error)"=w831) -> ("i ref out"=w829:refnum<vi>, "i attribute"=w827:T28, "error out"=w828:errorcluster)  [unwired: 15 in]
            n523 = Unbundle By Name(w827) -> ("Vision ID on same Node"=w826:string)
          }
        }
        n524 = call "PH_Interaction.Open or Create PCS Instances.vi"("System ID (N/A)"=w793, "Instance to create or open"=w794, "error IO"=w789) -> ("error out"=w797:errorcluster)  [unwired: 16 in]
      }
      event "PA-Backreflection-Meas", "fs_Synchrolock_Watch": Value Change {
        n525 = event-data() -> ("CtlRef"=w838:refnum<vi>, "OldVal"=w833:bool)  [unwired: 1 in]
        n526 = property class="Bool (strict)"(reference=w838, error in=w837, "Value"=w833) -> (error out=w840:errorcluster, "Label.Text"=w839:string)  [unwired: 1 out]
        n527 = call "PH_Interaction.Open or Create Singleton Instance.vi"("i ref in"=w834, "Instance to create or to open"=w839, "error IO"=w840) -> ("i ref out"=w835:refnum<vi>, "error out"=w836:errorcluster)  [unwired: 15 in]
      }
      event "\"D:\\PCS\\Remote Access\\ns.rdp\"", "\"D:\\PCS\\Remote Access\\fs.rdp\"", "\"D:\\PCS\\Remote Access\\PA-Input.rdp\"", "\"D:\\PCS\\Remote Access\\PA-Exit.rdp\"", "\"D:\\PCS\\Remote Access\\MA.rdp\"", "\"D:\\PCS\\Remote Access\\MA.rdp\" 2", "\"D:\\PCS\\Remote Access\\MAS.rdp\"", "\"D:\\PCS\\Remote Access\\COS.rdp\"", "\"D:\\PCS\\Remote Access\\Experiment.rdp\"", "\"D:\\PCS\\Remote Access\\Laserlabor.rdp\"", "\"D:\\PCS\\Remote Access\\uOPA.rdp\"": Value Change {
        n528 = event-data() -> ("CtlRef"=w855:refnum<vi>)  [unwired: 1 in]
        n529 = property class="Bool"(reference=w855, error in=w854) -> (error out=w841:errorcluster, "Label.Text"=w842:string)  [unwired: 1 out]
        n530 = Match Pattern(string=w842, regular expression=" 2") -> (before substring=w843:string, offset past match=w847:i32)  [unwired: 1 in, 2 out]
        n531 = Equal?(x=w847, y=-1) -> (x = y?=w845:bool)
        n532 = Select(t=w842, s=w845, f=w843) -> (s? t:f=w844:string)
        n533 = Concatenate Strings("mstsc " ("command line"), w844) -> (w850:string)
        n534 = call <vilib>:"System Exec.vi"("wait until completion? (T)"=FALSE, "error in (no error)"=w841, "command line"=w850) -> ("error out"=w852:errorcluster)  [unwired: 5 in, 3 out]
      }
      event User Event {
        n535 = event-data() -> ("Class"=w859:string)  [unwired: 1 in]
        n536 = call "PH_Beamline.set GUI Refs.vi"("i ref in"=w863, "Class"=w859, "PH Beamline GUI Refs"=w858, "PH_BL-Master GUI Refs"=w857, "System Information GUI Refs"=w856, "error in (no error)"=w862) -> ("i ref out"=w861:refnum<vi>, "error out"=w860:errorcluster)  [unwired: 12 in]
        n537 = call "PH_Class.set GUI Refs stored Occurence.vi"("i ref in"=w861, "error in (no error)"=w860) -> ("i ref out"=w864:refnum<vi>, "error out"=w865:errorcluster)  [unwired: 16 in]
      }
    }
  }
  "error out" <- w326
  n538 = property on="PA_Bypass_In" class="Pict (strict)"("Disabled"=w258) -> ()  [unwired: 2 in, 2 out]
  n539 = property on="PA_Bypass_Out" class="Pict (strict)"("Disabled"=w258) -> ()  [unwired: 2 in, 2 out]
  n540 = property on="PA_PC_WP_BB" class="Bool (strict)"("Disabled"=w258) -> ()  [unwired: 2 in, 2 out]
  n541 = property on="Shutter_Exp1" class="Bool (strict)"("Disabled"=w258) -> ()  [unwired: 2 in, 2 out]
  n542 = property on="Shutter_Exp2" class="Bool (strict)"("Disabled"=w258) -> ()  [unwired: 2 in, 2 out]
  n543 = property on="Shutter_Exp3" class="Bool (strict)"("Disabled"=w258) -> ()  [unwired: 2 in, 2 out]
  n544 = property on="Shutter_Exp4" class="Bool (strict)"("Disabled"=w258) -> ()  [unwired: 2 in, 2 out]
  n545 = property on="PA_PC_WP_2_BB" class="Bool (strict)"("Disabled"=w258) -> ()  [unwired: 2 in, 2 out]
  n546 = call "PH_Interaction.set PCS System.vi"() -> ("Enum"=w292:T31)  [unwired: 1 in]
  n547 = case shown="\"Laser\"" w292 {
    tunnel: ["" "Laser" "Vision" "Pulsed Power" "Special" "Beckhoff"] -> w291
    tunnel: [TRUE TRUE TRUE TRUE FALSE FALSE] -> w290
    tunnel: [u32 0 ("Color Box") u32 16776960 ("Color Box") u32 16711935 ("Color Box") u32 65535 ("Color Box") u32 16711680 ("Color Box") u32 16448250 ("Color Box")] -> w268
    frame "PCS", Default {
    }
    frame "Laser" {
    }
    frame "Vision" {
    }
    frame "PP" {
    }
    frame "Special" {
    }
    frame "Beckhoff" {
    }
  }
  n548 = property on="Image Statistician" class="Bool"("Visible"=w290) -> ()  [unwired: 2 in, 2 out]
  n549 = property on="PCS System Indicator" class="Bool (strict)"("Caption.Text"=w291, "Caption.TextColor"=w268) -> ()  [unwired: 2 in, 2 out]
  n550 = Unregister For Events(event registration refnum=w79) -> ()  [unwired: 1 in, 1 out]
  n551 = call "PH_Interaction.Super Destroy Me.vi"("i ref out"=w327) -> ()
